vi "Facade.vi"(0 "Data In":T7, 2 "Display State In":T4, 3 "Container State":T6) -> (6 "Data Out":T7, 7 "Display State Out":T4, 8 "Action":T3)   [LabVIEW 2017, in "3D Pie.xctl"]
uses:
  <vilib>/Math Plots/3D Math Plots/3D Pie/3D Pie XCtrl/3D Pie.xctl
  <vilib>/Math Plots/3D Math Plots/3D Pie/3D Pie XCtrl/Data.ctl
  <vilib>/Math Plots/3D Math Plots/3D Plot/3D Plot Datatype/3D Plot Datatype.lvclass
  <vilib>/_xctls/Container State.ctl
  <vilib>/Math Plots/3D Math Plots/3D Pie/3D Pie XCtrl/State.ctl
  <vilib>/Math Plots/3D Math Plots/3D Pie/3D Pie/3D Pie.lvclass
  e:/builds/penguin/labview/branches/2017/dev/dist/vi.lib/Math Plots/3D Math Plots/3D Plot/3D Plot/3D Plot.lvclass
  <vilib>/Math Plots/3D Math Plots/3D Plot/Action String/3DMathPlot Ctrl Act Queue.ctl
  <vilib>/Math Plots/3D Math Plots/3D Plot/Action String/3DMathPlot Ctrl Act Cluster.ctl
  <vilib>/Math Plots/3D Math Plots/3D Plot/Action String/3DMathPlot State Class.ctl
  <vilib>/_xctls/Action.ctl
  <vilib>/Math Plots/3D Math Plots/3D Plot/3D Plot/Typedef/Plot Action.ctl
  <vilib>/Math Plots/3D Math Plots/3D Plot/Action String/3DMathPlot Action String.ctl
  <vilib>/_xctls/XControlSupport.lvlib
  <vilib>/Math Plots/3D Math Plots/3D Plot/3D Plot/3D Plot.lvclass
panel:
  in  "Color Ramp Palette":T1 {"Active Plot" items=["Plot-1"]}
  out "3D Picture Control":refnum<vi>(3d-picture)
  out "Export Image":picture
  out "XY Graph":cluster{dbl, dbl}[](graph)
  out "Render Window":refnum<vi>
  in  "Projection Palette":T2
  out "Intensity Graph":dbl[][](graph)
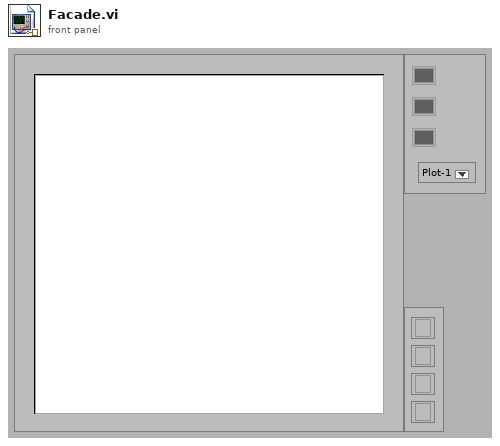
[diagram p1: front panel]
types:
  T1 = cluster{"Active Plot":i32, "Color Pair Array":cluster{"Color Box":u32, "String":string}[]}
  T2 = cluster{"XY Projection":bool, "XZ Projection":bool, "YZ Projection":bool, "3D Projection":bool}
  T3 = typedef "XControlSupport.lvlib/Action.ctl" = cluster{"Data Changed?":bool, "State Changed?":bool, "Action Name":string}
  T4 = typedef "3D Pie.xctl/State.ctl" = cluster{"3D Pie.lvclass":refnum<class "3D Pie.lvclass">, "Control Ref Queue":T5, "Plot Width":u32, "Main Frame Color":u32, "Ramp Palette Color":u32, "Projection Palette Color":u32}
  T5 = typedef "3DMathPlot Ctrl Act Queue.ctl" = refnum<queue>
  T6 = typedef "XControlSupport.lvlib/Container State.ctl" = cluster{"Indicator?":bool, "Run Mode?":bool, " Refnum":refnum<vi>}
  T7 = typedef "3D Pie.xctl/Data.ctl" = refnum<class "3D Plot Datatype.lvclass">[]
  T8 = typedef "3DMathPlot Ctrl Act Cluster.ctl" = cluster{"3D Picture Control":refnum<vi>, "Render Window Refnum":refnum<vi>, "XY Graph":refnum<vi>, "Intensity Graph":refnum<vi>, "Color Legend Palette":refnum<vi>, "Projection Palette":refnum<vi>, "XControl  Ref":refnum<vi>, "Facade Ref":refnum<vi>, "Export Image Ref":refnum<vi>, "Clear Data Flag":bool, "Display State Change Class":T9}
  T9 = typedef "3DMathPlot State Class.ctl" = enum16{"Update All Objects (Undo)", "Update Light Object Only", "Update Axis Object Only", "Update Plot Object Only", "Update Cursor Object Only", "Update Axis Plot Cursor Objects", "No Update"}
  T10 = typedef "3D Plot.lvclass/Actual Transform.ctl" = cluster{"Scale Cluster":cluster{"X Scale":sgl, "Y Scale":sgl, "Z Scale":sgl}, "Translate Cluster":cluster{"X Translate":sgl, "Y Translate":sgl, "Z Translate":sgl}, "Actual Range":T11}
  T11 = typedef "3D Plot.lvclass/Range Clusters.ctl" = cluster{"X Range":cluster{"Max X":sgl, "Min X":sgl}, "Y Range":cluster{"Max Y":sgl, "Min Y":sgl}, "Z Range":cluster{"Max Z":sgl, "Min Z":sgl}}
  T12 = typedef "3D Plot.lvclass/Plot Action.ctl" = cluster{"Light Action":enum16{"Update", "Remove", "Nothing"}, "Axis Action":enum16{"Update", "Remove", "Nothing"}, "Plot Action":enum16{"Update", "Remove", "Nothing"}, "Cursor Action":enum16{"Update", "Remove", "Nothing"}, "Fast Draw Action":enum16{"Update", "Remove", "Nothing"}}
  T13 = enum32{"Towards X-Y Plane", "Towards X-Z Plane", "Towards Y-Z Plane", "User Defined"}
  T14 = typedef "3D Plot.lvclass/Multiplot Representation.ctl" = cluster{"Plot Represention Array":T15[], "Max Range":T11}
  T15 = typedef "3D Plot.lvclass/Plot Representation.ctl" = cluster{"Plot ID":i32, "Plot Range":T11, "Mesh Data":T16, "Dimension":cluster{"X Dimension":i32, "Y Dimension":i32}, "Ramp Range":T11}
  T16 = typedef "3D Plot.lvclass/Mesh Data.ctl" = cluster{"Index Array":u32[], "Vertex Array":cluster{"X":sgl, "Y":sgl, "Z":sgl}[], "Normal Array":cluster{"X":sgl, "Y":sgl, "Z":sgl}[], "Color Index Array":i32[]}
  T17 = typedef "3D Plot.lvclass/Object Cluster.ctl" = cluster{"Root Scene Object":refnum<vi>, "Fast Root Scene Object":refnum<vi>}
  T18 = typedef "3DMathPlot Action String.ctl" = u16
  T19 = typedef "3D Plot.lvclass/Property Cluster.ctl" = cluster{"Graph Property":T20, "Light Property":T24, "Axis Property":T26, "Value Pair Property":T32, "Format Property":T34, "Cursor Property Array":T35, "Appearance Property":T44}
  T20 = typedef "3D Plot.lvclass/Graph Property.ctl" = cluster{"General Property":T21, "View Property":T22, "Grid Plane":T23}
  T21 = typedef "3D Plot.lvclass/General Property.ctl" = cluster{"Plot Area Color":u32, "Fast Draw?":bool, "Clip Data?":bool}
  T22 = typedef "3D Plot.lvclass/View Property.ctl" = cluster{"Projection Mode":enum16{"Orthographic", "Perspective"}, "View Direction":enum32{"Towards X-Y Plane", "Towards X-Z Plane", "Towards Y-Z Plane", "User Defined"}, "User Defined View Direction":cluster{"View Latitude":sgl, "View Longitude":sgl, "View Distance":sgl}}
  T23 = typedef "3D Plot.lvclass/Grid Plane.ctl" = cluster{"Grid Plane Visible":cluster{"Draw Grid Plane X-Y":bool, "Draw Grid Plane Y-Z":bool, "Draw Grid Plane X-Z":bool}, "Grid Antialiasing":bool, "Grid Frame Color":u32}
  T24 = typedef "3D Plot.lvclass/Light Property.ctl" = cluster{"Enable Lighting?":bool, "Ambient Color":u32, "Light Array":T25[]}
  T25 = typedef "3D Plot.lvclass/Light Specific.ctl" = cluster{"Enable Light?":bool, "Light Color":u32, "Light Latitude":sgl, "Light Longitude":sgl, "Light Distance":sgl, "Attenuation":enum16{"None", "Linear", "Quadratic"}}
  T26 = typedef "3D Plot.lvclass/Axis Property.ctl" = cluster{"Caption Property":T27, "Label Property":T28, "Range Property":T29, "Grid Property":T30, "Ticks Property":T31}
  T27 = typedef "3D Plot.lvclass/Caption Property.ctl" = cluster{"Show Caption":cluster{"Show Normal X Caption":bool, "Show Normal Y Caption":bool, "Show Normal Z Caption":bool, "Show Opposite X Caption":bool, "Show Opposite Y Caption":bool, "Show Opposite Z Caption":bool}, "Caption Color":cluster{"Caption Color X":u32, "Caption Color Y":u32, "Caption Color Z":u32}, "Caption Size":cluster{"Caption Size X":u16, "Caption Size Y":u16, "Caption Size Z":u16}, "Caption String":cluster{"Caption X":string, "Caption Y":string, "Caption Z ":string}}
  T28 = typedef "3D Plot.lvclass/Label Property.ctl" = cluster{"Show Label":cluster{"Show Normal X Label":bool, "Show Normal Y Label":bool, "Show Normal Z Label":bool, "Show Opposite X Label":bool, "Show Opposite Y Label":bool, "Show Opposite Z Label":bool}, "Label Color":cluster{"Label Color X":u32, "Label Color Y":u32, "Label Color Z":u32}, "Label Size":cluster{"Label Size X":u16, "Label Size Y":u16, "Labe Size Z":u16}}
  T29 = typedef "3D Plot.lvclass/Range Property.ctl" = cluster{"Range Cluster":T11, "Auto Range":cluster{"Auto Range X":bool, "Auto Range Y":bool, "Auto Range Z":bool}, "Inverted":cluster{"Inverted X":bool, "Inverted Y":bool, "Inverted Z":bool}, "Logarithm":cluster{"Logarithm X":bool, "Logarithm Y":bool, "Logarithm Z":bool}}
  T30 = typedef "3D Plot.lvclass/Grid Property.ctl" = cluster{"Major Grid Visible":cluster{"Draw Major Grid X":bool, "Draw Major Grid Y":bool, "Draw Major Grid Z":bool}, "Major Grid Color":cluster{"Major Grid Color X":u32, "Major Grid Color Y":u32, "Major Grid Color Z":u32}, "Minor Grid Visible":cluster{"Draw Minor Grid X":bool, "Draw Minor Grid Y":bool, "Draw Minor Grid Z":bool}, "Minor Grid Color":cluster{"Minor Grid Color X":u32, "Minor Grid Color Y":u32, "Minor Grid Color Z":u32}}
  T31 = typedef "3D Plot.lvclass/Tick Property.ctl" = cluster{"Major Tick Visible":cluster{"Draw Major Tick X":bool, "Draw Major Tick Y":bool, "Draw Major Tick Z":bool}, "Major Tick Color":cluster{"Major Tick Color X":u32, "Major Tick Color Y":u32, "Major Tick Color Z":u32}, "Major Count":cluster{"Major Count X":u16, "Major Count Y":u16, "Major Count Z":u16}, "Minor Tick Visible":cluster{"Draw Minor Tick X":bool, "Draw Minor Tick Y":bool, "Draw Minor Tick Z":bool}, "Minor Tick Color":cluster{"Minor Tick Color X":u32, "Minor Tick Color Y":u32, "Minor Tick Color Z":u32}, "Minor Count":cluster{"Minor Count X":u16, "Minor Count Y":u16, "Minor Count Z":u16}}
  T32 = typedef "3D Plot.lvclass/Value Pair Property.ctl" = T33[]
  T33 = typedef "3D Plot.lvclass/Value Pair Cluster.ctl" = cluster{"Value Pair Array":cluster{"Value":sgl, "Name":string}[], "Show Tick":bool, "Show Grid":bool, " Label Mode":enum16{"Name", "Value", "None"}}
  T34 = typedef "3D Plot.lvclass/Format Property.ctl" = string[]
  T35 = typedef "3D Plot.lvclass/Cursor Property Array.ctl" = T36[]
  T36 = typedef "3D Plot.lvclass/Cursor Property.ctl" = cluster{"Cursor Visible":bool, "Cursor Enable":bool, "Cursor Position":T37, "Cursor Point":T38, "Cursor Line":T40, "Cursor Plane":T42, "Cursor Text":T43}
  T37 = typedef "3D Plot.lvclass/Cursor Position.ctl" = cluster{"Cursor Plot ID":i32, "Cursor X":sgl, "Cursor Y":sgl, "Cursor Z":sgl, "Cursor Snap To":enum16{"Fixed", "Nearest Plot", "Snap to Plot"}}
  T38 = typedef "3D Plot.lvclass/Cursor Point.ctl" = cluster{"Cursor Point Color":u32, "Cursor Point Size":sgl, "Cursor Point Style":T39}
  T39 = typedef "3D Plot.lvclass/Sprite Type.ctl" = enum16{"None", "Empty Square", "Solid Square", "Empty Diamond", "Solid Diamond", "Empty Circle", "Solid Circle", "Asterisk", "Bold X", "Wireframe Sphere", "Solid Sphere", "Wireframe Cube", "Solid Cube"}
  T40 = typedef "3D Plot.lvclass/Cursor Line.ctl" = cluster{"Cursor Line Color":u32, "Cursor Line Width":sgl, "Cursor Line Style":T41}
  T41 = typedef "3D Plot.lvclass/Line Type.ctl" = enum16{"None", "Solid", "Dash", "Dot", "Dash Dot"}
  T42 = typedef "3D Plot.lvclass/Cursor Plane.ctl" = cluster{"Cursor Plane Color":u32, "Cursor Plane Opacity":sgl, "Draw Cursor Plane X-Z":bool, "Draw Cursor Plane Y-Z":bool, "Draw Cursor Plane X-Y":bool}
  T43 = typedef "3D Plot.lvclass/Cursor Text.ctl" = cluster{"Cursor Text":string, "Cursor Text Size":u16, "Cursor Show Position":bool, "Cursor Show Name":bool, "Cursor Text Color":u32, "Background Color":u32, "Background Opacity":sgl}
  T44 = typedef "3D Plot.lvclass/Apearance Property.ctl" = cluster{"Visibility":T45, "Active Index":cluster{"Active Plot":i32, "Active Cursor":i32, "Active Axis":enum16{"X-axis", "Y-axis", "Z-axis"}, "Active Value Pair":enum16{"X-axis", "Y-axis", "Z-axis"}, "Active Light":enum16{"Light 0", "Light 1", "Light 2", "Light 3"}}, "Backup Data":cluster{"Plot Name":string[]}}
  T45 = typedef "3D Plot.lvclass/Item Visibility.ctl" = cluster{"Projection Palette":bool, "Color Ramp Palette":bool}
  T46 = typedef "LVPoint32TypeDef.ctl" = cluster{"Horizontal":i32, "Vertical":i32}
  T47 = typedef "LVRangeTypeDef.ctl" = cluster{"Minimum":dbl, "Maximum":dbl, "Increment":dbl, "Minor Increment":dbl, "Start":dbl}
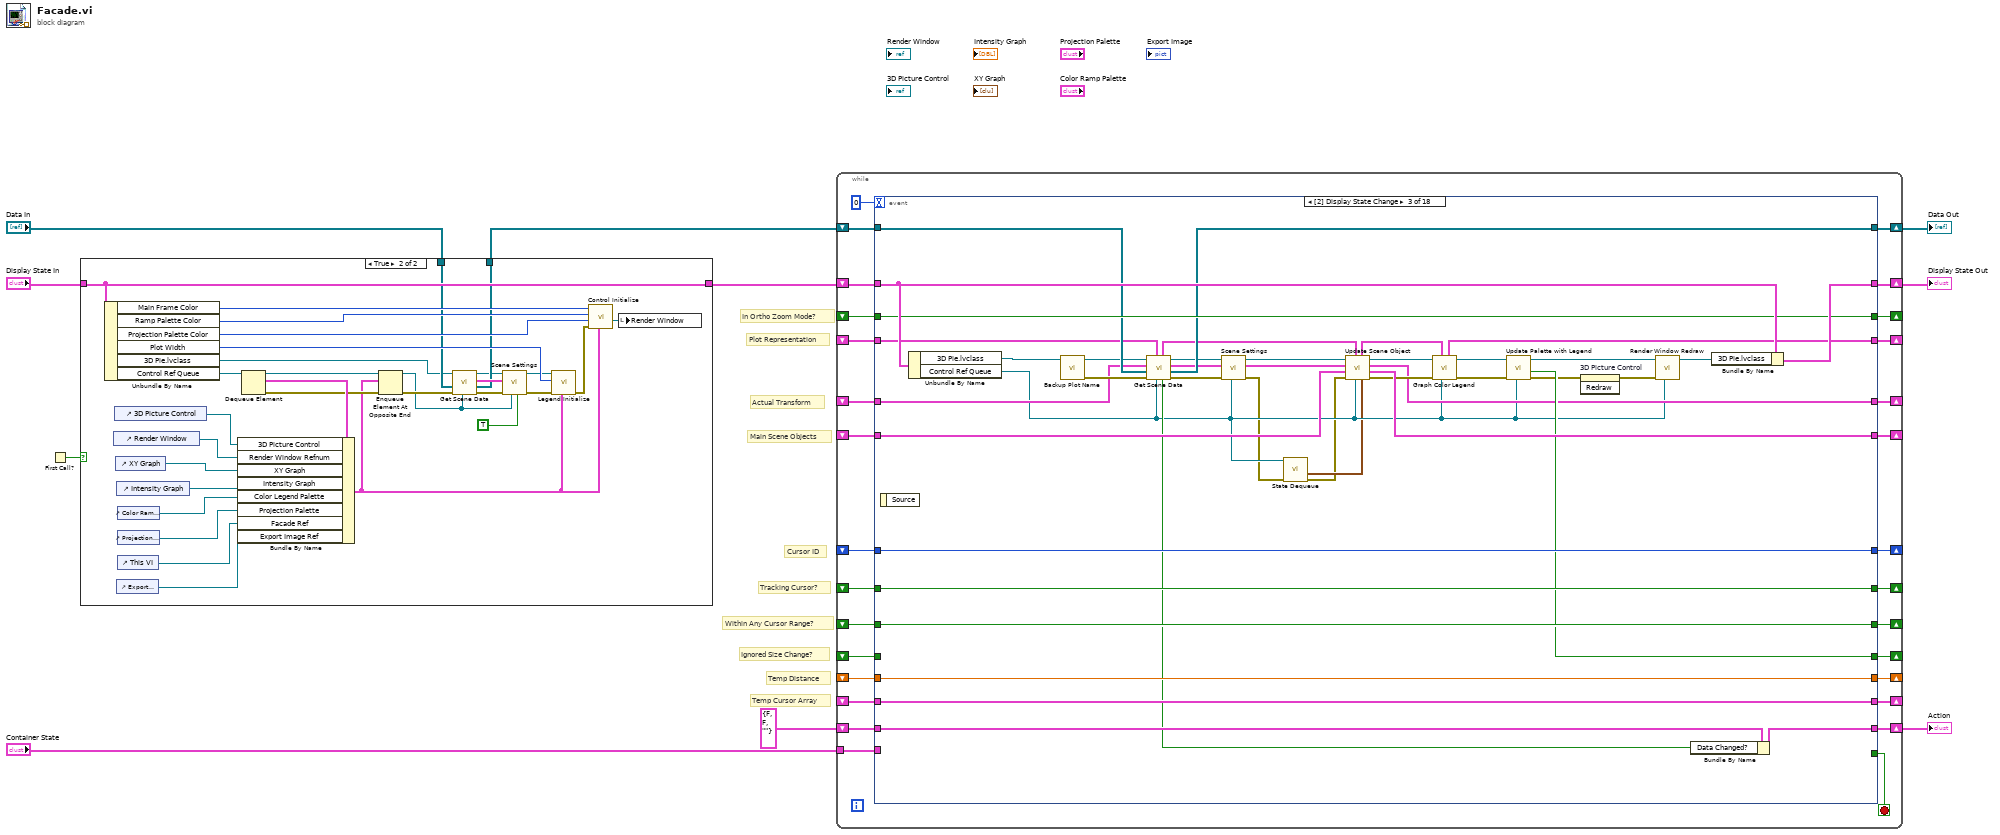
[diagram p0: block diagram]
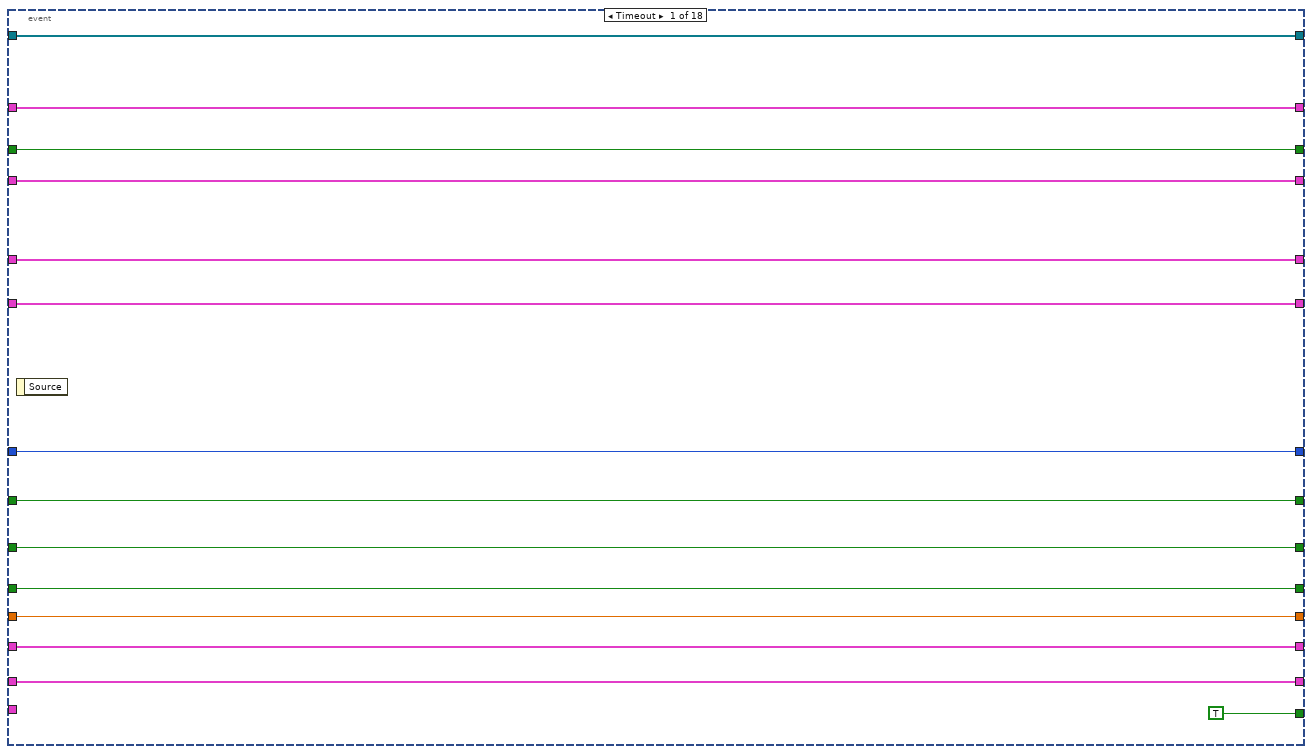
[diagram p2: hidden frame]
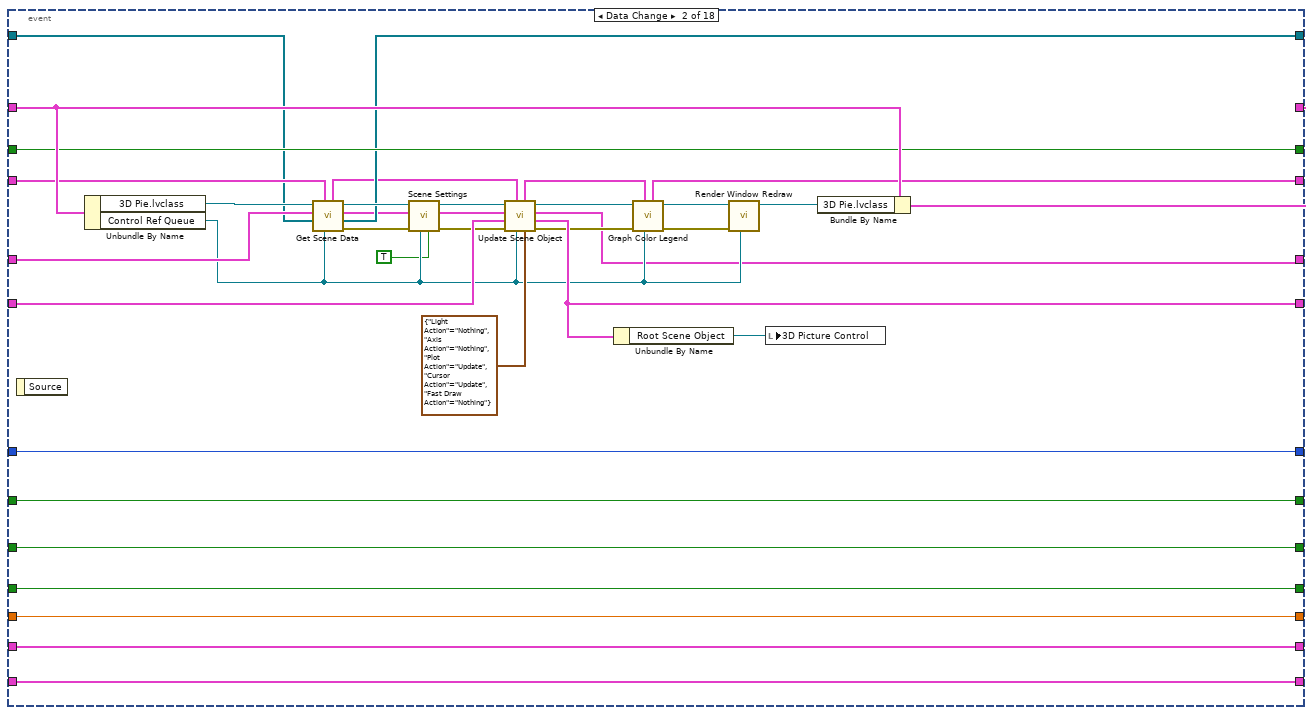
[diagram p3: hidden frame]
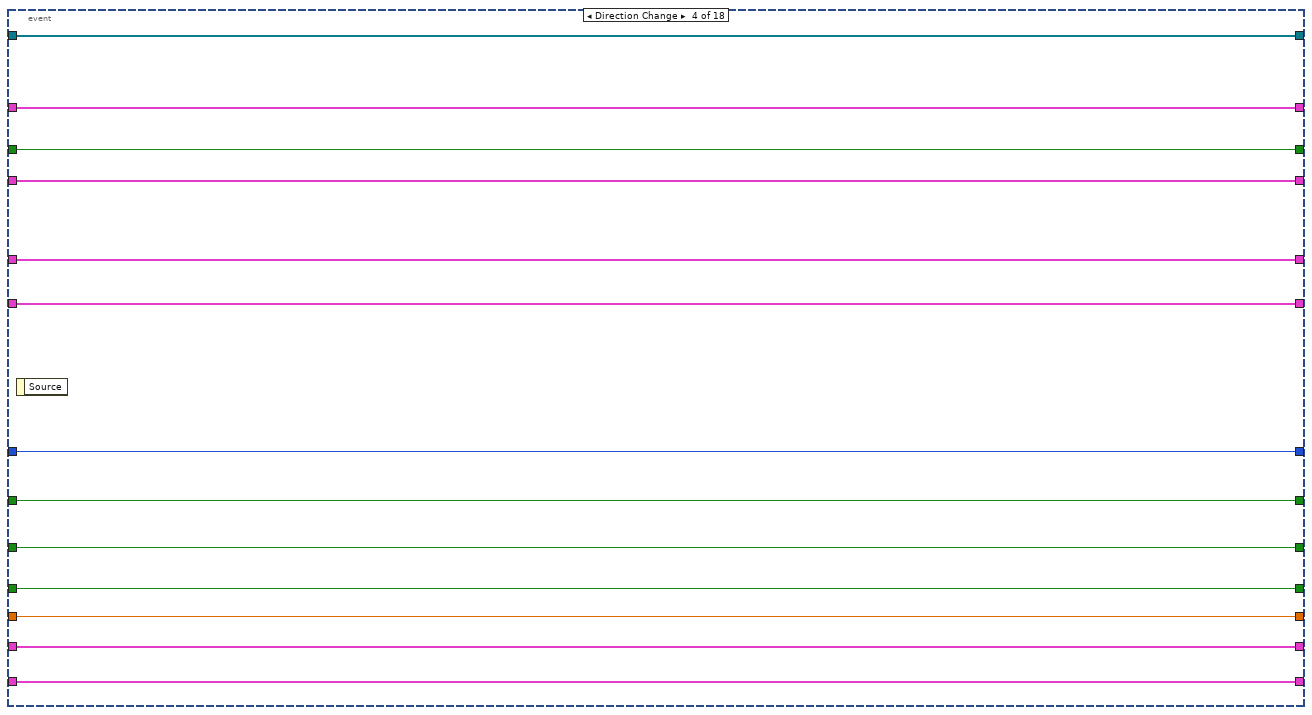
[diagram p4: hidden frame]
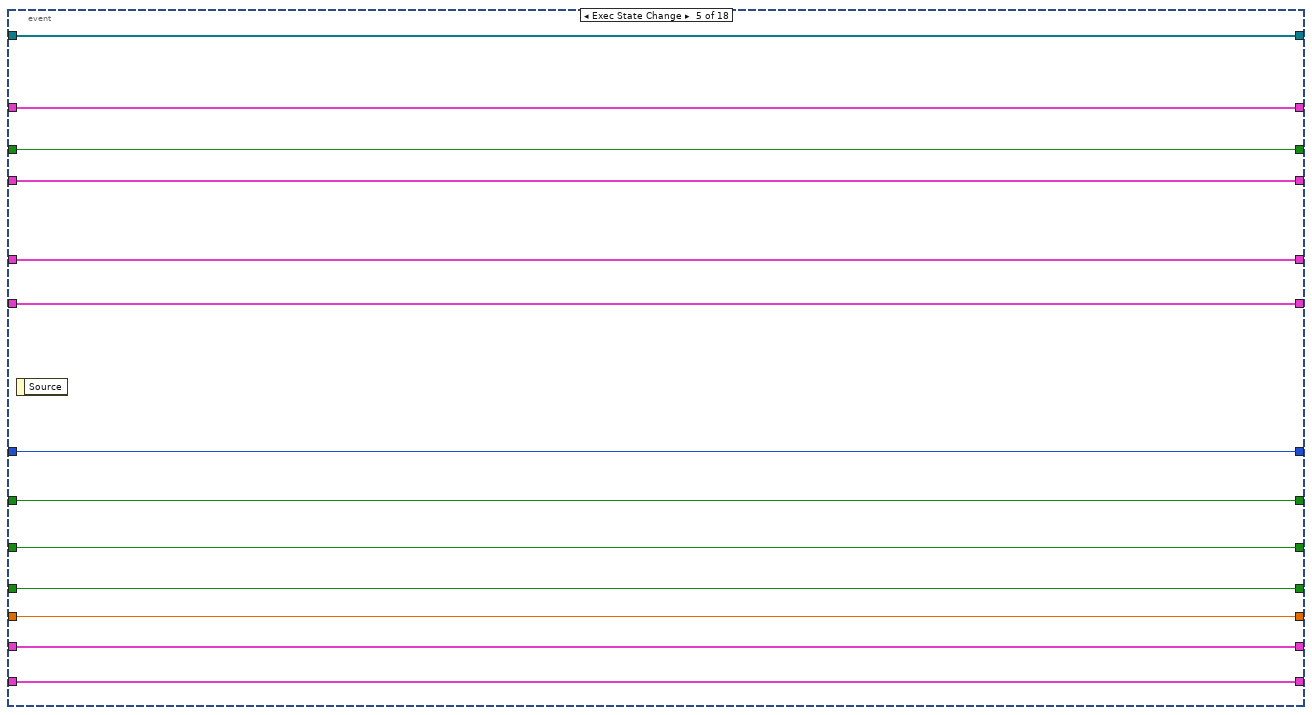
[diagram p5: hidden frame]
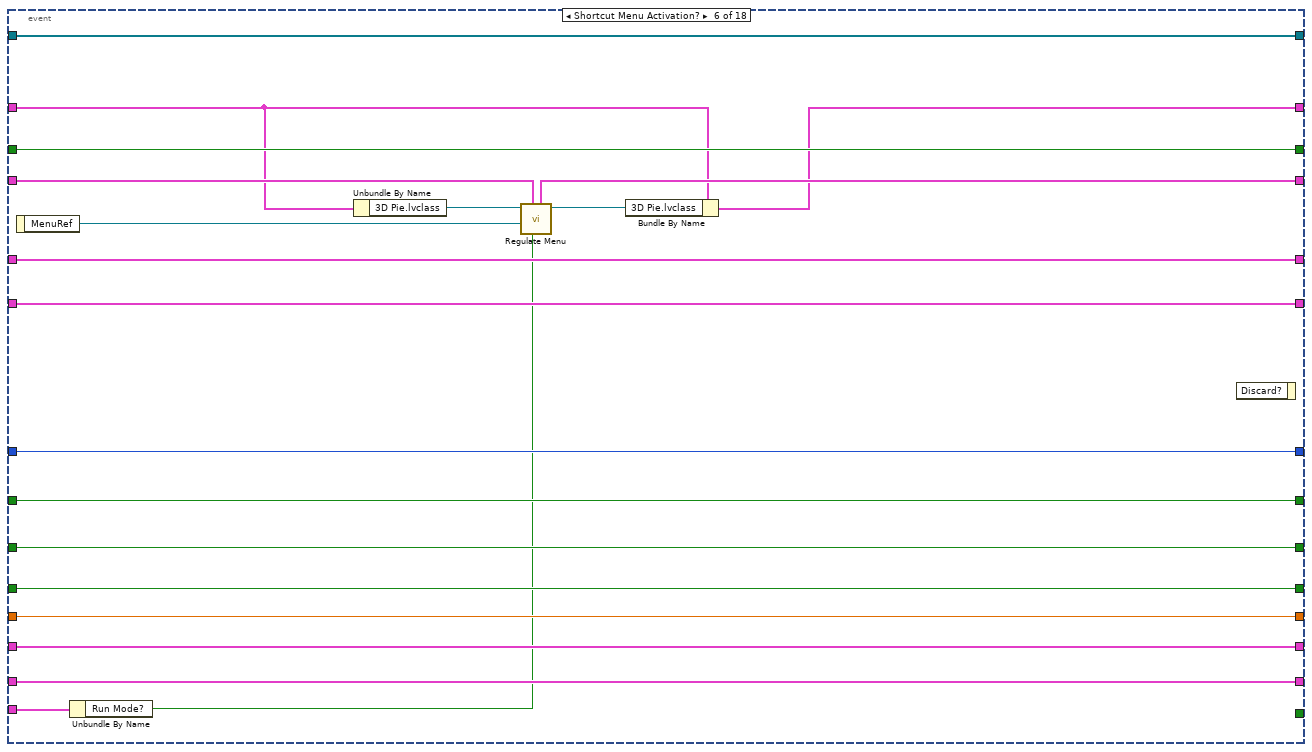
[diagram p6: hidden frame]
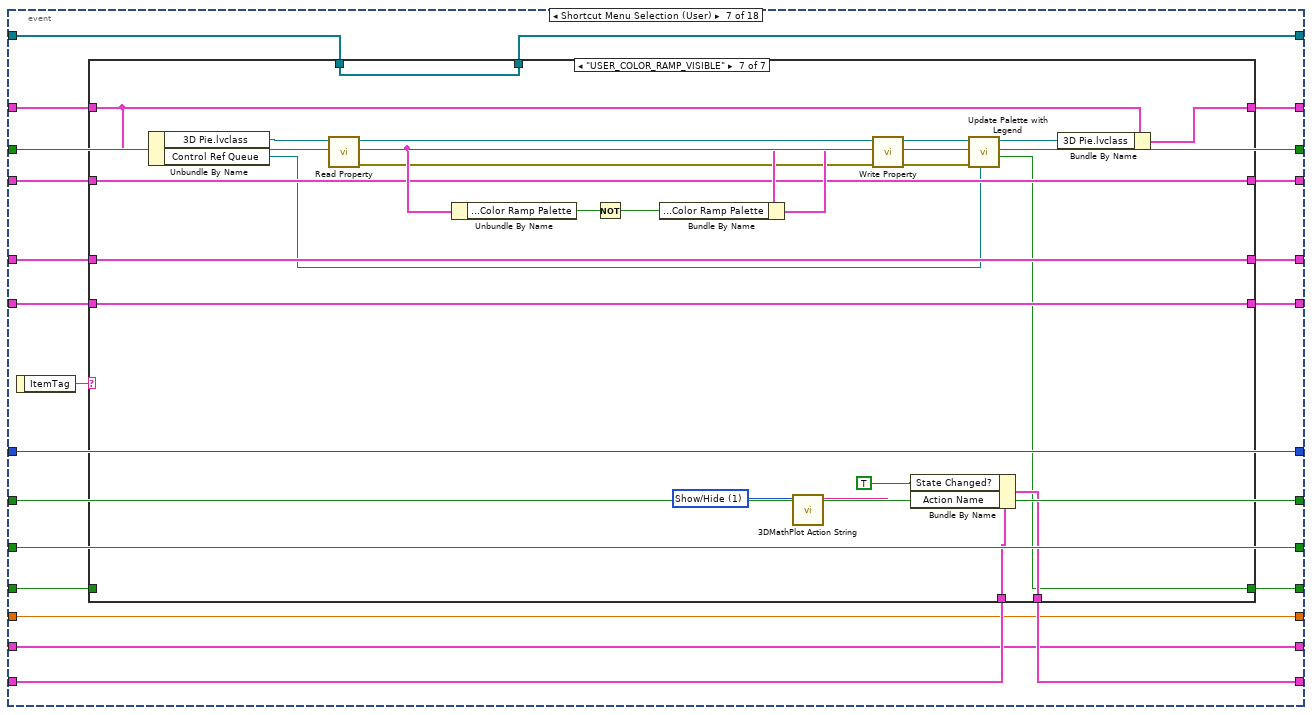
[diagram p7: hidden frame]
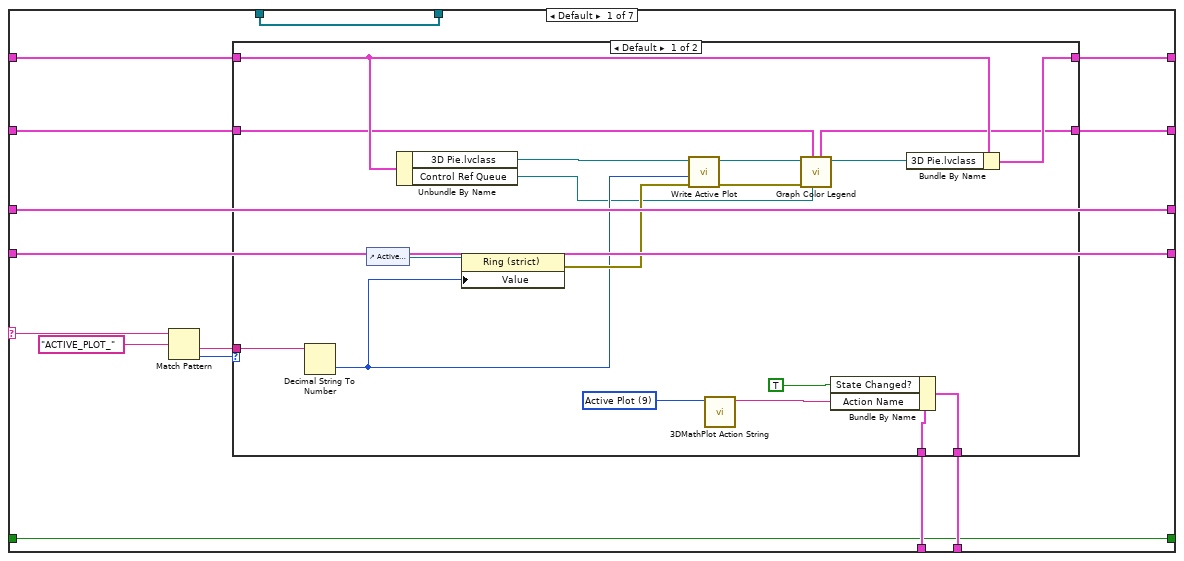
[diagram p8: hidden frame]
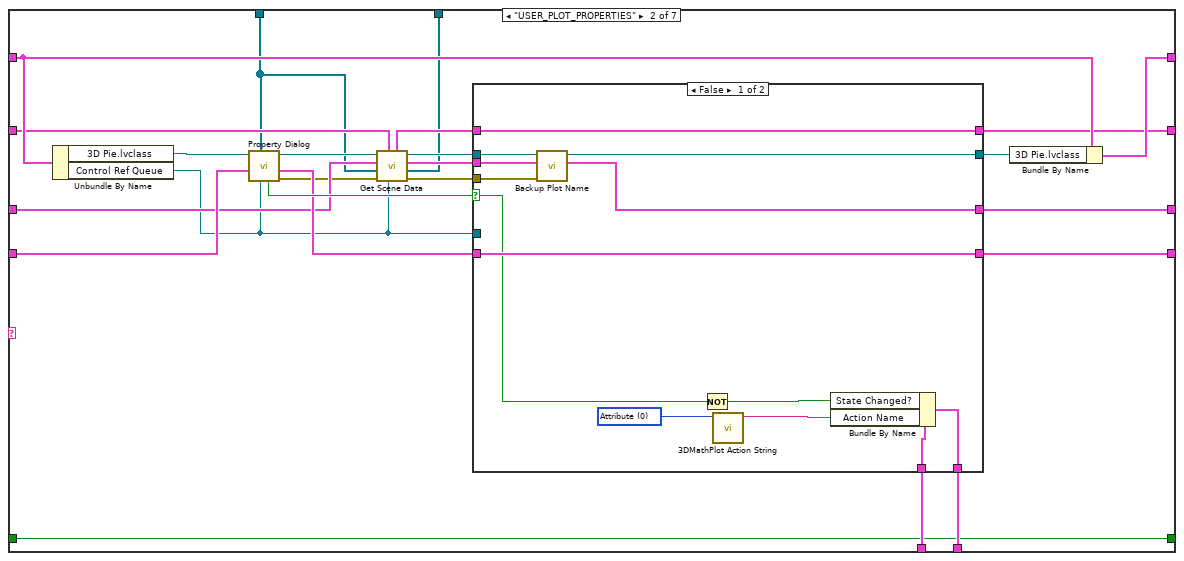
[diagram p10: hidden frame]
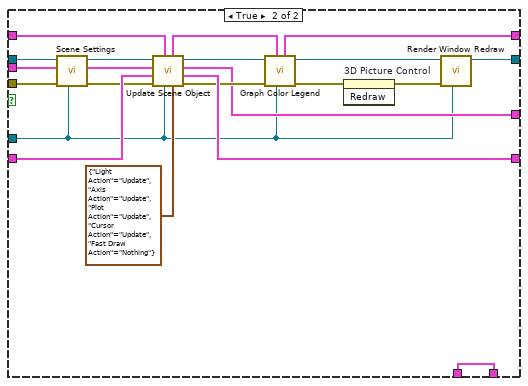
[diagram p11: hidden frame]
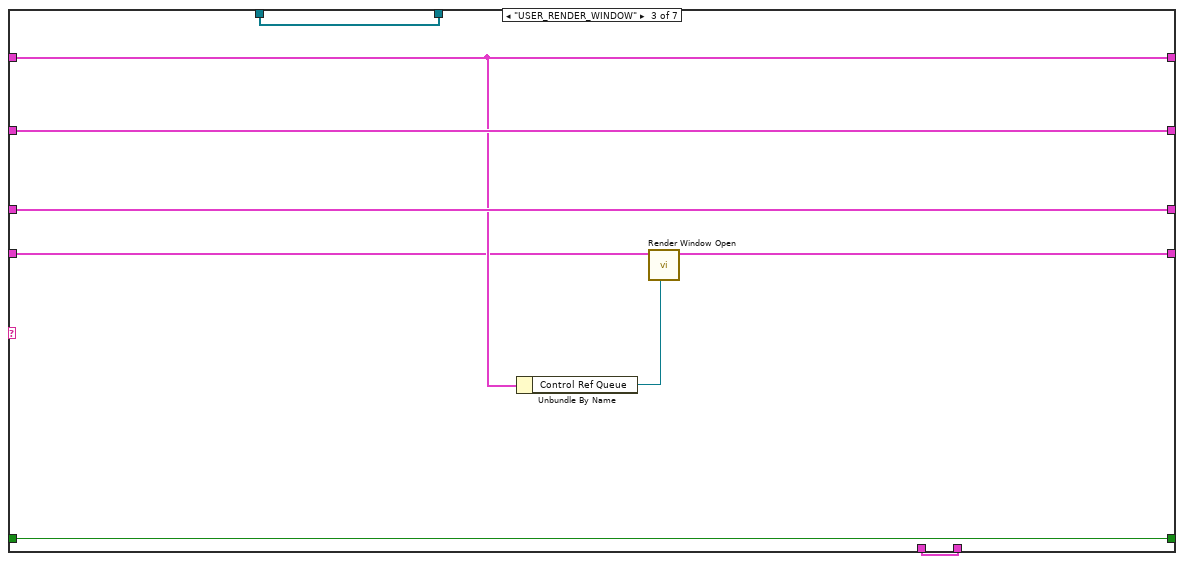
[diagram p12: hidden frame]
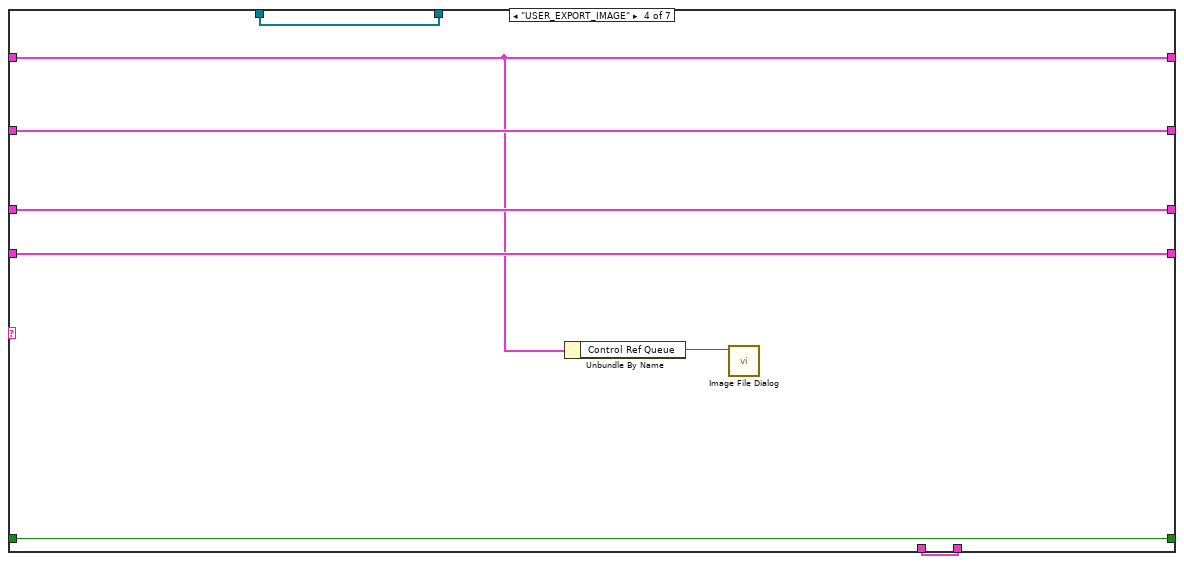
[diagram p13: hidden frame]
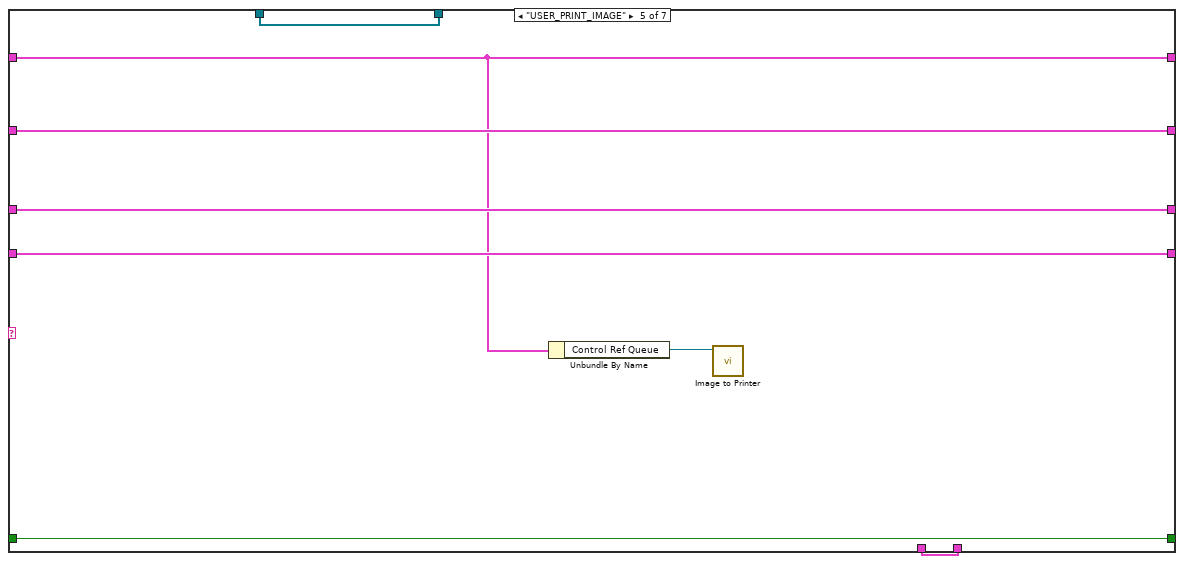
[diagram p14: hidden frame]
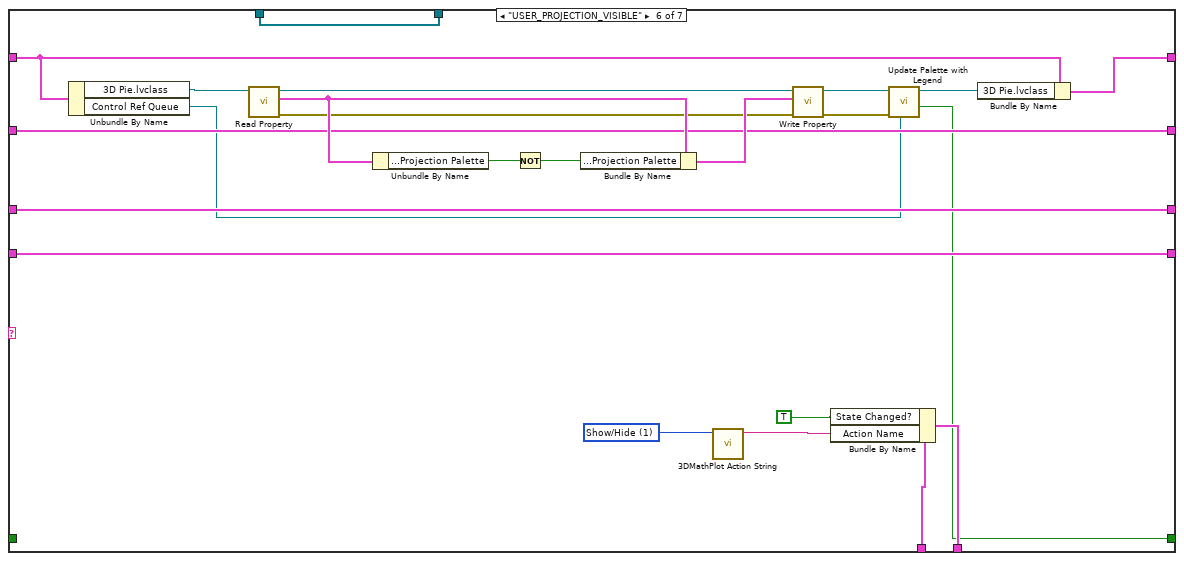
[diagram p15: hidden frame]
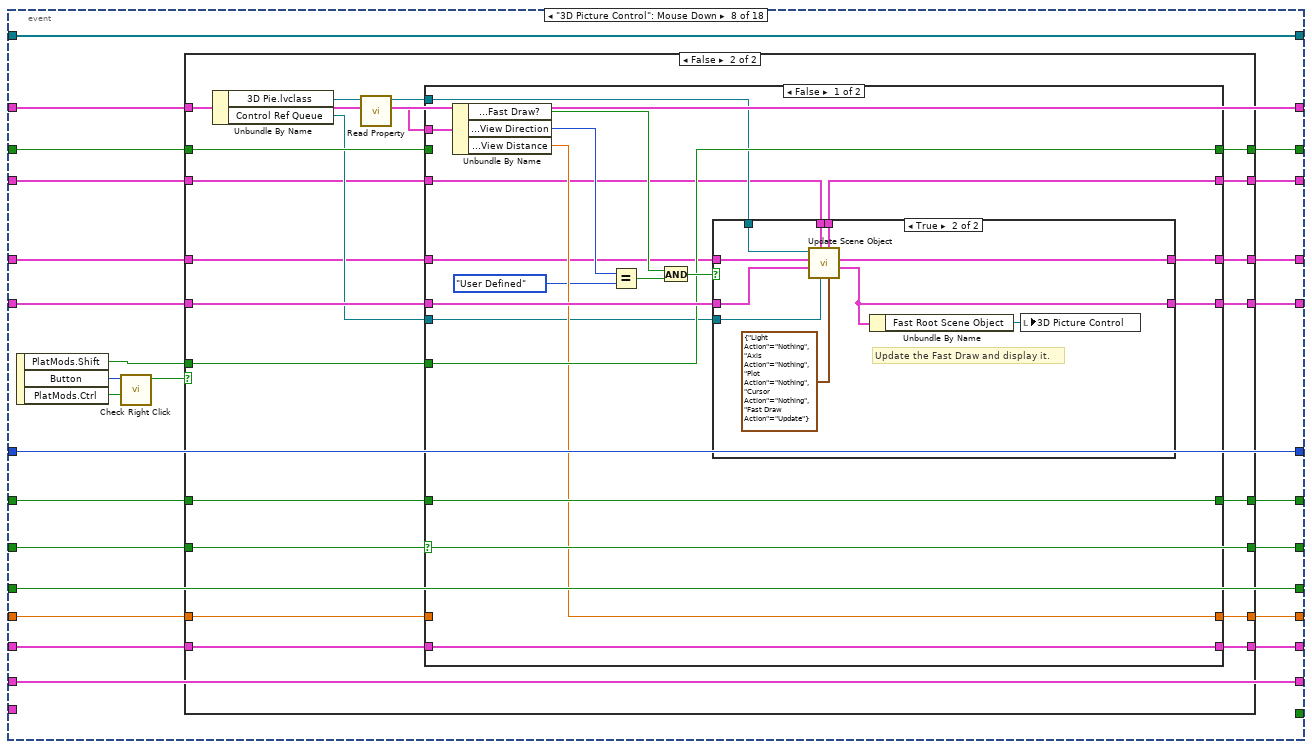
[diagram p16: hidden frame]
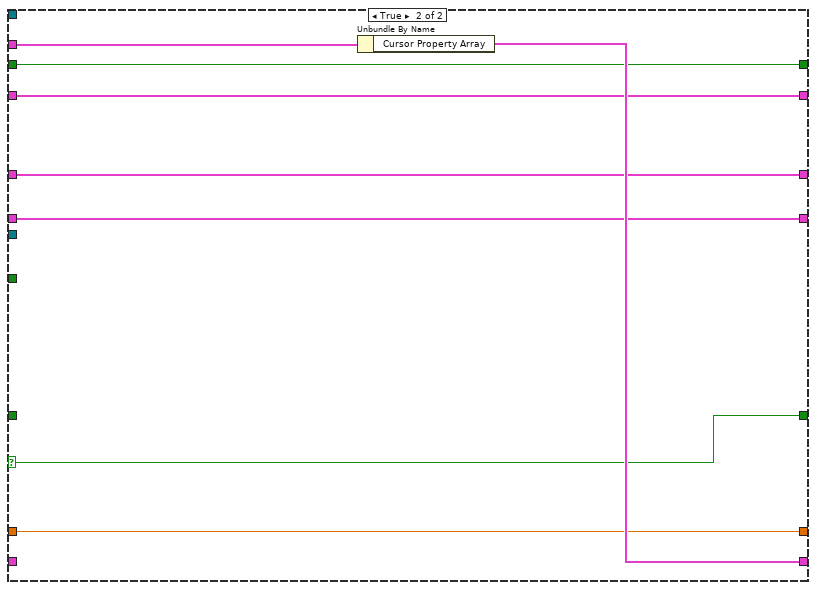
[diagram p19: hidden frame]
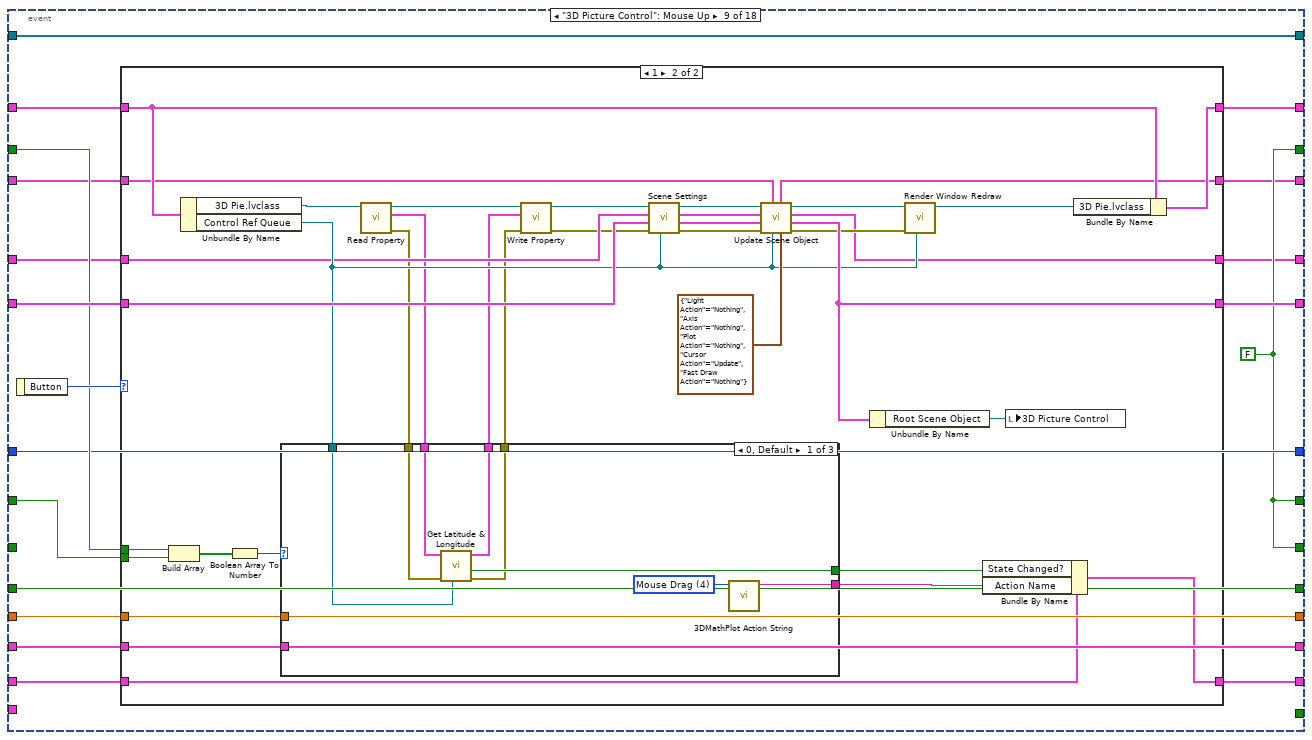
[diagram p20: hidden frame]
diagram:
  # "Ignored Size Change?"
  # "Actual Transform"
  # "Temp Cursor Array"
  # "Temp Distance"
  # "Within Any Cursor Range?"
  # "Tracking Cursor?"
  # "Cursor ID"
  # "Plot Representation"
  # "In Ortho Zoom Mode?"
  # "Main Scene Objects"
  n1 = First Call?() -> (First Call?: T/F=w10:bool)
  n2 = case shown="True" w10 {
    tunnel: "Display State In" -> [w12 w32]
    tunnel: [w12 w32] -> w8
    tunnel: "Data In" -> [w11 w18]
    tunnel: [w11 w17] -> w1
    frame False {
    }
    frame True {
      n3 = Unbundle By Name(w32) -> ("Main Frame Color"=w27:u32, "Ramp Palette Color"=w26:u32, "Projection Palette Color"=w25:u32, "Plot Width"=w23:u32, "3D Pie.lvclass"=w16:refnum<class "3D Pie.lvclass">, "Control Ref Queue"=w31:T5)
      n4 = control-ref of="Render Window"() -> (w37:refnum<vi>)
      n5 = control-ref of="3D Picture Control"() -> (w38:refnum<vi>)
      n6 = control-ref of="XY Graph"() -> (w36:refnum<vi>)
      n7 = control-ref of="Intensity Graph"() -> (w35:refnum<vi>)
      n8 = control-ref of="Export Image"() -> (w30:refnum<vi>)
      n9 = control-ref of="Color Ramp Palette"() -> (w34:refnum<vi>)
      n10 = control-ref of="Projection Palette"() -> (w33:refnum<vi>)
      n11 = control-ref of="This VI"() -> (w42:refnum<vi>)
      n12 = Dequeue Element(queue=w31) -> (queue out=w40:T5, element=w41:T8, error out=w39:errorcluster)  [unwired: 1 in, 2 out]
      n13 = Bundle By Name(cluster=w41, "3D Picture Control"=w38, "Render Window Refnum"=w37, "XY Graph"=w36, "Intensity Graph"=w35, "Color Legend Palette"=w34, "Projection Palette"=w33, "Facade Ref"=w42, "Export Image Ref"=w30) -> (w28:T8)
      n14 = Enqueue Element At Opposite End(queue=w40, element=w28, error in (no error)=w39) -> (queue out=w20:T5, error out=w22:errorcluster)  [unwired: 2 out]
      n15 = call <vilib>:"Get Scene Data.vi"("Control Ref Queue"=w20, "error in (no error)"=w22, "Data In"=w18, "3D Plot.lvclass in"=w16) -> ("error out"=w13:errorcluster, "Data Out"=w17:refnum<class "3D Plot Datatype.lvclass">[], "Actual Transform Out"=w24:T10, "3D Plot.lvclass out"=w15:refnum<class "3D Pie.lvclass">)  [unwired: 2 in, 2 out]
      n16 = call <vilib>:"Scene Settings.vi"("Data Change Event?"=TRUE, "Control Ref Queue"=w20, "error in (no error)"=w13, "Actual Transform In"=w24, "3D Plot.lvclass in"=w15) -> ("error out"=w21:errorcluster, "3D Plot.lvclass out"=w14:refnum<class "3D Pie.lvclass">)  [unwired: 2 in, 3 out]
      n17 = call <vilib>:"Legend Initialize.vi"("Control Ref Cluster"=w28, "error in (no error)"=w21, "XY Plot Width"=w23, "3D Plot.lvclass"=w14) -> ("error out"=w29:errorcluster)  [unwired: 7 out]
      n18 = call <vilib>:"Control Initialize.vi"("Control Ref Cluster"=w28, "error in (no error)"=w29, "Projection Palette Color"=w25, "Ramp Palette Color"=w26, "Main Frame Color"=w27) -> ("New Window Refnum"=w43:refnum<vi>)  [unwired: 6 out]
      n19 = local write "Render Window"(w43) -> ()
    }
  }
  n20 = while {
    shift-right: [w71] -> w4
    shift-left: w8 -> [w72]
    tunnel: "Container State" -> [w68]
    shift-right: [w67] -> w5
    shift-left: w1 -> [w62]
    shift-right: [w65] -> w3
    shift-left: T3 {"Data Changed?"=FALSE, "State Changed?"=FALSE, "Action Name"=""} ("Action") -> [w66]
    shift-right: [w64] -> _
    shift-left: _ -> [w63]
    shift-right: [w61] -> _
    shift-left: _ -> [w48]
    shift-right: [w59] -> _
    shift-left: _ -> [w60]
    shift-right: [w58] -> _
    shift-left: _ -> [w57]
    shift-right: [w55] -> _
    shift-left: _ -> [w56]
    shift-right: [w54] -> _
    shift-left: _ -> [w53]
    shift-right: [w52] -> _
    shift-left: _ -> [w51]
    shift-right: [w50] -> _
    shift-left: _ -> [w49]
    shift-right: [w47] -> _
    shift-left: _ -> [w46]
    shift-right: [w45] -> _
    shift-left: _ -> [w44]
    stop <- w70 stop-if-true
    n21 = event shown="[2] Display State Change" {
      selector: _ -> [_ _ _ _ _ _ _ _ _ _ _ _ _ _ _ _ _ _]
      dyn-events: _ -> [_ _ _ _ _ _ _ _ _ _ _ _ _ _ _ _ _ _]
      timeout: 0 -> [_ _ _ _ _ _ _ _ _ _ _ _ _ _ _ _ _ _]
      tunnel: w72 -> [w74 w121 w161 w175 w188 w190 w225 w407 w500 w583 w609 w636 w663 w690 w714 w737 w800 w818]
      tunnel: [w74 w120 w160 w175 w188 w189 w224 w407 w497 w583 w606 w635 w662 w689 w713 w732 w799 w817] -> w71
      tunnel: [TRUE _ _ _ _ _ _ _ _ _ _ _ _ _ _ _ _ _] -> w70
      tunnel: w68 -> [_ _ _ _ _ w198 _ _ _ _ _ _ _ _ _ _ _ _]
      tunnel: w62 -> [w84 w96 w151 w174 w187 w208 w213 w416 w503 w587 w615 w642 w669 w696 w721 w722 w809 w826]
      tunnel: [w84 w95 w152 w174 w187 w208 w212 w416 w503 w587 w615 w642 w669 w696 w721 w722 w809 w826] -> w67
      tunnel: [w85 w111 w140 w173 w186 w206 w226 w415 w498 w586 w607 w633 w660 w687 w707 w735 w796 w824] -> w65
      tunnel: w66 -> [w85 w111 w162 w173 w186 w206 w227 w415 w499 w586 w608 w634 w661 w688 w708 w734 w797 w824]
      tunnel: [w76 w110 w154 w172 w185 w207 w228 w402 w501 w580 w599 w627 w653 w681 w702 w733 w795 w825] -> w64
      tunnel: w63 -> [w76 w113 w155 w172 w185 w207 w229 w411 w502 w581 w599 w627 w653 w681 w702 w738 w794 w825]
      tunnel: [w83 w118 w153 w171 w184 w205 w218 w399 w491 w584 w610 w641 w668 w695 w720 w743 w804 w821] -> w61
      tunnel: w48 -> [w83 w118 w153 w171 w184 w205 w218 w408 w495 w585 w610 w641 w668 w695 w720 w743 w804 w821]
      tunnel: w60 -> [w82 w117 w159 w170 w183 w204 w219 w414 w492 w579 w611 w640 w667 w694 w719 w729 w805 w822]
      tunnel: [w82 w117 w159 w170 w183 w204 w219 w414 w492 w578 w611 w640 w667 w694 w719 w729 w805 w822] -> w59
      tunnel: w57 -> [w81 w116 w158 w169 w182 w203 w220 w406 w494 w575 w612 w639 w666 w693 w718 w728 w806 w823]
      tunnel: [w81 w116 w158 w169 w182 w203 w220 w398 w491 w575 w612 w639 w666 w693 w718 w728 w806 w823] -> w58
      tunnel: w56 -> [w80 w115 w157 w168 w181 w202 w221 w405 _ _ w613 w638 w665 w692 w717 w727 w807 w819]
      tunnel: [w80 w115 w157 w168 w181 w202 w221 w397 w491 w574 w613 w638 w665 w692 w717 w727 w807 w819] -> w55
      tunnel: [w79 w114 w156 w167 w180 w201 w222 w395 w493 w577 w614 w637 w664 w691 w716 w723 w808 w820] -> w54
      tunnel: w53 -> [w79 w114 w156 w167 w180 w201 w222 w403 w493 _ w614 w637 w664 w691 w716 w723 w808 w820]
      tunnel: [w77 w89 w127 w166 w179 w193 w216 w400 w489 w573 w591 w624 w651 w678 w697 w731 w782 w814] -> w52
      tunnel: w51 -> [w77 w98 w133 w166 w179 w194 w217 w409 w490 w573 w591 w624 w651 w678 w698 w736 w778 w814]
      tunnel: w49 -> [w78 w97 w134 w165 w178 w200 w215 w410 w488 w572 w593 w623 w650 w677 w703 w740 w781 w815]
      tunnel: [w78 w88 w128 w165 w178 w200 w214 w401 w487 w572 w592 w622 w649 w676 w703 w730 w783 w815] -> w50
      tunnel: [w75 w107 w147 w164 w177 w199 w211 w413 w486 w571 w603 w630 w657 w684 w705 w724 w791 FALSE] -> w47
      tunnel: w46 -> [w75 w107 _ w164 w177 w199 w210 w413 w486 w571 w603 w630 w657 w684 w705 w726 w791 w811]
      tunnel: [w73 w101 w141 w163 w176 w197 w209 w396 w485 w565 w601 w628 w655 w682 w701 w725 w784 w813] -> w45
      tunnel: w44 -> [w73 w101 w141 w163 w176 w197 w209 w404 w485 _ w601 w628 w655 w682 w701 w725 w784 w813]
      event Timeout {
        n22 = event-data() -> ()  [unwired: 2 out]
      }
      event Data Change {
        n23 = event-data() -> ()  [unwired: 2 out]
        n24 = Unbundle By Name(w121) -> ("3D Pie.lvclass"=w100:refnum<class "3D Pie.lvclass">, "Control Ref Queue"=w92:T5)
        n25 = call <vilib>:"Get Scene Data.vi"("Control Ref Queue"=w92, "Multiplot Representation In"=w98, "Data In"=w96, "Actual Transform In"=w97, "3D Plot.lvclass in"=w100) -> ("error out"=w93:errorcluster, "Data Out"=w95:refnum<class "3D Plot Datatype.lvclass">[], "Actual Transform Out"=w94:T10, "3D Plot.lvclass out"=w99:refnum<class "3D Pie.lvclass">, "Multiplot Representation Out"=w91:T14)  [unwired: 1 in, 1 out]
        n26 = call <vilib>:"Scene Settings.vi"("Data Change Event?"=TRUE, "Control Ref Queue"=w92, "error in (no error)"=w93, "Actual Transform In"=w94, "3D Plot.lvclass in"=w99) -> ("error out"=w102:errorcluster, "Actual Transform Out"=w112:T10, "3D Plot.lvclass out"=w103:refnum<class "3D Pie.lvclass">)  [unwired: 2 in, 2 out]
        n27 = call <vilib>:"Update Scene Object.vi"("Action"=T12 {"Light Action"=enum."Nothing", "Axis Action"=enum."Nothing", "Plot Action"=enum."Update", "Cursor Action"=enum."Update", "Fast Draw Action"=enum."Nothing"}, "Control Ref Queue"=w92, "Multiplot Representation In"=w91, "error in (no error)"=w102, "Object Cluster In"=w113, "Actual Transform In"=w112, "3D Plot.lvclass in"=w103) -> ("error out"=w108:errorcluster, "Object Cluster Out"=w110:T17, "Actual Transform Out"=w88:T10, "3D Plot.lvclass out"=w109:refnum<class "3D Pie.lvclass">, "Multiplot Representation Out"=w90:T14)
        n28 = Unbundle By Name(w110) -> ("Root Scene Object"=w119:refnum<vi>)
        n29 = call-dynamic "Graph Color Legend.vi"("Control Ref Queue"=w92, "Multiplot Representation In"=w90, "error in (no error)"=w108, "3D Pie.lvclass in"=w109) -> ("error out"=w104:errorcluster, "3D Pie.lvclass out"=w105:refnum<class "3D Pie.lvclass">, "Multiplot Representation Out"=w89:T14)  [unwired: 2 in, 3 out]
        n30 = call <vilib>:"Render Window Redraw.vi"("Control Ref Queue"=w92, "error in (no error)"=w104) -> ()  [unwired: 1 in, 9 out]
        n31 = local write "3D Picture Control"(w119) -> ()
        n32 = Bundle By Name(cluster=w121, "3D Pie.lvclass"=w105) -> (w120:T4)
      }
      event Display State Change {
        n33 = event-data() -> ()  [unwired: 2 out]
        n34 = Unbundle By Name(w161) -> ("3D Pie.lvclass"=w126:refnum<class "3D Pie.lvclass">, "Control Ref Queue"=w125:T5)
        n35 = call-dynamic "Backup Plot Name.vi"("3D Pie.lvclass in"=w126) -> ("error out"=w135:errorcluster, "3D Pie.lvclass out"=w138:refnum<class "3D Pie.lvclass">)  [unwired: 1 in, 8 out]
        n36 = call <vilib>:"Get Scene Data.vi"("Control Ref Queue"=w125, "Multiplot Representation In"=w133, "error in (no error)"=w135, "Data In"=w151, "Actual Transform In"=w134, "3D Plot.lvclass in"=w138) -> ("error out"=w137:errorcluster, "Data Out"=w152:refnum<class "3D Plot Datatype.lvclass">[], "Actual Transform Out"=w132:T10, "3D Plot.lvclass out"=w136:refnum<class "3D Pie.lvclass">, "Data Cleaned?"=w139:bool, "Multiplot Representation Out"=w130:T14)
        n37 = call <vilib>:"Scene Settings.vi"("Control Ref Queue"=w125, "error in (no error)"=w137, "Actual Transform In"=w132, "3D Plot.lvclass in"=w136) -> ("error out"=w122:errorcluster, "Actual Transform Out"=w131:T10, "3D Plot.lvclass out"=w142:refnum<class "3D Pie.lvclass">)  [unwired: 3 in, 2 out]
        n38 = call <vilib>:"State Dequeue.vi"("error in (no error)"=w122, "Control Ref Queue"=w125) -> ("error out"=w123:errorcluster, "Action"=w124:T12)  [unwired: 8 out]
        n39 = call <vilib>:"Update Scene Object.vi"("Action"=w124, "Control Ref Queue"=w125, "Multiplot Representation In"=w130, "error in (no error)"=w123, "Object Cluster In"=w155, "Actual Transform In"=w131, "3D Plot.lvclass in"=w142) -> ("error out"=w149:errorcluster, "Object Cluster Out"=w154:T17, "Actual Transform Out"=w128:T10, "3D Plot.lvclass out"=w150:refnum<class "3D Pie.lvclass">, "Multiplot Representation Out"=w129:T14)
        n40 = call-dynamic "Graph Color Legend.vi"("Control Ref Queue"=w125, "Multiplot Representation In"=w129, "error in (no error)"=w149, "3D Pie.lvclass in"=w150) -> ("error out"=w145:errorcluster, "3D Pie.lvclass out"=w146:refnum<class "3D Pie.lvclass">, "Multiplot Representation Out"=w127:T14)  [unwired: 2 in, 3 out]
        n41 = call <vilib>:"Update Palette with Legend.vi"("Control Ref Queue"=w125, "error in (no error)"=w145, "3D Plot.lvclass"=w146) -> ("error out"=w144:errorcluster, "Ignore the size change?"=w147:bool, "3D Plot.lvclass out"=w148:refnum<class "3D Pie.lvclass">)  [unwired: 6 out]
        n42 = invoke on="3D Picture Control" class="SceneGraphDisp (strict)" method="Redraw"(error in=w144) -> (error out=w143:errorcluster)  [unwired: 2 in, 2 out]
        n43 = call <vilib>:"Render Window Redraw.vi"("Control Ref Queue"=w125, "error in (no error)"=w143) -> ()  [unwired: 1 in, 9 out]
        n44 = Bundle By Name(cluster=w162, "Data Changed?"=w139) -> (w140:T3)
        n45 = Bundle By Name(cluster=w161, "3D Pie.lvclass"=w148) -> (w160:T4)
      }
      event Direction Change {
        n46 = event-data() -> ()  [unwired: 2 out]
      }
      event Exec State Change {
        n47 = event-data() -> ()  [unwired: 2 out]
      }
      event Shortcut Menu Activation? {
        n48 = event-data() -> ("MenuRef"=w192:refnum<k9>)  [unwired: 1 out]
        n49 = Unbundle By Name(w198) -> ("Run Mode?"=w191:bool)
        n50 = Unbundle By Name(w190) -> ("3D Pie.lvclass"=w196:refnum<class "3D Pie.lvclass">)
        n51 = call <vilib>:"Regulate Menu.vi"("Run Mode?"=w191, "Multiplot Representation In"=w194, "MenuRef"=w192, "3D Plot.lvclass in"=w196) -> ("3D Plot.lvclass out"=w195:refnum<class "3D Pie.lvclass">, "Multiplot Representation Out"=w193:T14)  [unwired: 3 in, 3 out]
        n52 = Bundle By Name(cluster=w190, "3D Pie.lvclass"=w195) -> (w189:T4)
        n53 = event-data() -> ()  [unwired: 1 in, 2 out]
      }
      event Shortcut Menu Selection (User) {
        n54 = event-data() -> ("ItemTag"=w223:string)  [unwired: 1 out]
        n55 = case shown="\"USER_COLOR_RAMP_VISIBLE\"" w223 {
          selector: w223 -> [w242 _ _ _ _ _ _]
          tunnel: w225 -> [w239 w288 w324 w331 w338 w359 w385]
          tunnel: [w238 w287 w324 w331 w338 w358 w384] -> w224
          tunnel: w229 -> [w243 w278 w322 w337 w345 w364 w383]
          tunnel: [w243 w285 w321 w337 w345 w364 w383] -> w228
          tunnel: w227 -> [w235 w281 w327 w336 w340 w367 w380]
          tunnel: [w236 w280 w327 w336 w340 w366 w379] -> w226
          tunnel: w217 -> [w232 w273 w328 w335 w344 w357 w382]
          tunnel: [w231 w284 w328 w335 w344 w357 w382] -> w216
          tunnel: w215 -> [w230 w271 w325 w332 w343 w356 w381]
          tunnel: [w230 w282 w325 w332 w343 w356 w381] -> w214
          tunnel: w213 -> [w234 w269 w329 w334 w342 w353 w376]
          tunnel: [w234 w268 w329 w334 w342 w353 w376] -> w212
          tunnel: [w233 w279 w326 w333 w339 w347 w370] -> w211
          tunnel: w210 -> [w233 w279 w326 w333 w339 _ _]
          frame Default {
            n56 = Match Pattern(string=w242, regular expression="ACTIVE_PLOT_") -> (after substring=w237:string, offset past match=w240:i32)  [unwired: 3 out]
            n57 = case shown="Default" w240 {
              tunnel: w239 -> [w254 w264]
              tunnel: [w253 w264] -> w238
              tunnel: w237 -> [w260 _]
              tunnel: [w255 w263] -> w236
              tunnel: w235 -> [w256 w263]
              tunnel: w232 -> [w246 w262]
              tunnel: [w245 w262] -> w231
              frame Default {
                w257 = T18 9 items=["Attribute", "Show/Hide", "Cursor Move", "Zoom", "Mouse Drag", "XY Projection", "YZ Projection", "XZ Projection", "3D Projection", "Active Plot", "Scale"] ("Global String")
                n58 = Decimal String To Number(string=w260) -> (number=w251:i32)  [unwired: 3 out]
                n59 = control-ref of="Active Plot"() -> (w244:refnum<vi>)
                n60 = Unbundle By Name(w254) -> ("3D Pie.lvclass"=w261:refnum<class "3D Pie.lvclass">, "Control Ref Queue"=w249:T5)
                n61 = property class="Ring (strict)"(reference=w244, "Value"=w251) -> (error out=w252:errorcluster)  [unwired: 1 in, 1 out]
                n62 = call-dynamic "Write Active Plot.vi"("error in (no error)"=w252, "Active Plot"=w251, "3D Plot.lvclass in"=w261) -> ("error out"=w247:errorcluster, "3D Plot.lvclass out"=w248:refnum<class "3D Pie.lvclass">)  [unwired: 7 in]
                n63 = call <vilib>:"3DMathPlot Action String.vi"("Global String"=w257) -> ("String Out"=w258:string)  [unwired: 10 out]
                n64 = call-dynamic "Graph Color Legend.vi"("Control Ref Queue"=w249, "Multiplot Representation In"=w246, "error in (no error)"=w247, "3D Pie.lvclass in"=w248) -> ("3D Pie.lvclass out"=w250:refnum<class "3D Pie.lvclass">, "Multiplot Representation Out"=w245:T14)  [unwired: 2 in, 4 out]
                n65 = Bundle By Name(cluster=w256, "State Changed?"=TRUE ("Data Changed?"), "Action Name"=w258) -> (w255:T3)
                n66 = Bundle By Name(cluster=w254, "3D Pie.lvclass"=w250) -> (w253:T4)
              }
              frame -1 {
              }
            }
          }
          frame "USER_PLOT_PROPERTIES" {
            n67 = Unbundle By Name(w288) -> ("3D Pie.lvclass"=w286:refnum<class "3D Pie.lvclass">, "Control Ref Queue"=w265:T5)
            n68 = call-dynamic "Property Dialog.vi"("Control Ref Queue"=w265, "Data"=w269, "Object Cluster In"=w278, "3D Pie in"=w286) -> ("error out"=w267:errorcluster, "Object Cluster Out"=w276:T17, "3D Pie out"=w275:refnum<class "3D Pie.lvclass">, "Cancel?"=w277:bool)  [unwired: 1 in, 3 out]
            n69 = call <vilib>:"Get Scene Data.vi"("Control Ref Queue"=w265, "Multiplot Representation In"=w273, "error in (no error)"=w267, "Data In"=w269, "Actual Transform In"=w271, "3D Plot.lvclass in"=w275) -> ("error out"=w266:errorcluster, "Data Out"=w268:refnum<class "3D Plot Datatype.lvclass">[], "Actual Transform Out"=w270:T10, "3D Plot.lvclass out"=w274:refnum<class "3D Pie.lvclass">, "Multiplot Representation Out"=w272:T14)  [unwired: 1 out]
            n70 = case shown="False" w277 {
              selector: w277 -> [w290 _]
              tunnel: w276 -> [w298 w313]
              tunnel: w272 -> [w299 w304]
              tunnel: [w298 w320] -> w285
              tunnel: [w299 w307] -> w284
              tunnel: w274 -> [w293 w302]
              tunnel: w266 -> [w292 w303]
              tunnel: [w291 w317] -> w283
              tunnel: [w300 w306] -> w282
              tunnel: w270 -> [w300 w301]
              tunnel: w281 -> [w295 w314]
              tunnel: [w294 w314] -> w280
              tunnel: w265 -> [_ w305]
              frame False {
                w296 = T18 0 items=["Attribute", "Show/Hide", "Cursor Move", "Zoom", "Mouse Drag", "XY Projection", "YZ Projection", "XZ Projection", "3D Projection", "Active Plot", "Scale"] ("Global String")
                n71 = call-dynamic "Backup Plot Name.vi"("error in (no error)"=w292, "3D Pie.lvclass in"=w293) -> ("3D Pie.lvclass out"=w291:refnum<class "3D Pie.lvclass">)  [unwired: 9 out]
                n72 = Not(x=w290) -> (.not. x?=w289:bool)
                n73 = call <vilib>:"3DMathPlot Action String.vi"("Global String"=w296) -> ("String Out"=w297:string)  [unwired: 10 out]
                n74 = Bundle By Name(cluster=w295, "State Changed?"=w289, "Action Name"=w297) -> (w294:T3)
              }
              frame True {
                n75 = call <vilib>:"Scene Settings.vi"("Control Ref Queue"=w305, "error in (no error)"=w303, "Actual Transform In"=w301, "3D Plot.lvclass in"=w302) -> ("error out"=w309:errorcluster, "Actual Transform Out"=w319:T10, "3D Plot.lvclass out"=w310:refnum<class "3D Pie.lvclass">)  [unwired: 3 in, 2 out]
                n76 = call <vilib>:"Update Scene Object.vi"("Action"=T12 {"Light Action"=enum."Update", "Axis Action"=enum."Update", "Plot Action"=enum."Update", "Cursor Action"=enum."Update", "Fast Draw Action"=enum."Nothing"}, "Control Ref Queue"=w305, "Multiplot Representation In"=w304, "error in (no error)"=w309, "Object Cluster In"=w313, "Actual Transform In"=w319, "3D Plot.lvclass in"=w310) -> ("error out"=w316:errorcluster, "Object Cluster Out"=w320:T17, "Actual Transform Out"=w306:T10, "3D Plot.lvclass out"=w318:refnum<class "3D Pie.lvclass">, "Multiplot Representation Out"=w308:T14)
                n77 = call-dynamic "Graph Color Legend.vi"("Control Ref Queue"=w305, "Multiplot Representation In"=w308, "error in (no error)"=w316, "3D Pie.lvclass in"=w318) -> ("error out"=w312:errorcluster, "3D Pie.lvclass out"=w317:refnum<class "3D Pie.lvclass">, "Multiplot Representation Out"=w307:T14)  [unwired: 2 in, 3 out]
                n78 = invoke on="3D Picture Control" class="SceneGraphDisp (strict)" method="Redraw"(error in=w312) -> (error out=w311:errorcluster)  [unwired: 2 in, 2 out]
                n79 = call <vilib>:"Render Window Redraw.vi"("Control Ref Queue"=w305, "error in (no error)"=w311) -> ()  [unwired: 1 in, 9 out]
              }
            }
            n80 = Bundle By Name(cluster=w288, "3D Pie.lvclass"=w283) -> (w287:T4)
          }
          frame "USER_RENDER_WINDOW" {
            n81 = Unbundle By Name(w324) -> ("Control Ref Queue"=w323:T5)
            n82 = call <vilib>:"Render Window Open.vi"("Control Ref Queue"=w323, "Object Cluster In"=w322) -> ("Object Cluster Out"=w321:T17)  [unwired: 3 in, 6 out]
          }
          frame "USER_EXPORT_IMAGE" {
            n83 = Unbundle By Name(w331) -> ("Control Ref Queue"=w330:T5)
            n84 = call <vilib>:"Image File Dialog.vi"("Control Ref Queue"=w330) -> ()  [unwired: 2 in, 9 out]
          }
          frame "USER_PRINT_IMAGE" {
            n85 = Unbundle By Name(w338) -> ("Control Ref Queue"=w341:T5)
            n86 = call <vilib>:"Image to Printer.vi"("Control Ref Queue"=w341) -> ()  [unwired: 1 in, 10 out]
          }
          frame "USER_PROJECTION_VISIBLE" {
            w355 = T18 1 items=["Attribute", "Show/Hide", "Cursor Move", "Zoom", "Mouse Drag", "XY Projection", "YZ Projection", "XZ Projection", "3D Projection", "Active Plot", "Scale"] ("Global String")
            n87 = Unbundle By Name(w359) -> ("3D Pie.lvclass"=w363:refnum<class "3D Pie.lvclass">, "Control Ref Queue"=w346:T5)
            n88 = call <vilib>:"Read Property.vi"("3D Plot.lvclass in"=w363) -> ("error out"=w348:errorcluster, "Property Cluster"=w361:T19, "3D Plot.lvclass out"=w362:refnum<class "3D Pie.lvclass">)  [unwired: 1 in, 7 out]
            n89 = Unbundle By Name(w361) -> ("Appearance Property.Visibility.Projection Palette"=w365:bool)
            n90 = Not(x=w365) -> (.not. x?=w352:bool)
            n91 = Bundle By Name(cluster=w361, "Appearance Property.Visibility.Projection Palette"=w352) -> (w360:T19)
            n92 = call <vilib>:"3DMathPlot Action String.vi"("Global String"=w355) -> ("String Out"=w354:string)  [unwired: 10 out]
            n93 = call <vilib>:"Write Property.vi"("error in (no error)"=w348, "Property Cluster"=w360, "3D Plot.lvclass in"=w362) -> ("error out"=w351:errorcluster, "3D Plot.lvclass out"=w350:refnum<class "3D Pie.lvclass">)  [unwired: 7 out]
            n94 = Bundle By Name(cluster=w367, "State Changed?"=TRUE ("Data Changed?"), "Action Name"=w354) -> (w366:T3)
            n95 = call <vilib>:"Update Palette with Legend.vi"("Control Ref Queue"=w346, "error in (no error)"=w351, "3D Plot.lvclass"=w350) -> ("Ignore the size change?"=w347:bool, "3D Plot.lvclass out"=w349:refnum<class "3D Pie.lvclass">)  [unwired: 7 out]
            n96 = Bundle By Name(cluster=w359, "3D Pie.lvclass"=w349) -> (w358:T4)
          }
          frame "USER_COLOR_RAMP_VISIBLE" {
            w377 = T18 1 items=["Attribute", "Show/Hide", "Cursor Move", "Zoom", "Mouse Drag", "XY Projection", "YZ Projection", "XZ Projection", "3D Projection", "Active Plot", "Scale"] ("Global String")
            n97 = Unbundle By Name(w385) -> ("3D Pie.lvclass"=w389:refnum<class "3D Pie.lvclass">, "Control Ref Queue"=w369:T5)
            n98 = call <vilib>:"Read Property.vi"("3D Plot.lvclass in"=w389) -> ("error out"=w371:errorcluster, "Property Cluster"=w388:T19, "3D Plot.lvclass out"=w375:refnum<class "3D Pie.lvclass">)  [unwired: 1 in, 7 out]
            n99 = Unbundle By Name(w388) -> ("Appearance Property.Visibility.Color Ramp Palette"=w390:bool)
            n100 = Not(x=w390) -> (.not. x?=w378:bool)
            n101 = Bundle By Name(cluster=w388, "Appearance Property.Visibility.Color Ramp Palette"=w378) -> (w387:T19)
            n102 = call <vilib>:"3DMathPlot Action String.vi"("Global String"=w377) -> ("String Out"=w386:string)  [unwired: 10 out]
            n103 = call <vilib>:"Write Property.vi"("error in (no error)"=w371, "Property Cluster"=w387, "3D Plot.lvclass in"=w375) -> ("error out"=w374:errorcluster, "3D Plot.lvclass out"=w373:refnum<class "3D Pie.lvclass">)  [unwired: 7 out]
            n104 = Bundle By Name(cluster=w380, "State Changed?"=TRUE ("Data Changed?"), "Action Name"=w386) -> (w379:T3)
            n105 = call <vilib>:"Update Palette with Legend.vi"("Control Ref Queue"=w369, "error in (no error)"=w374, "3D Plot.lvclass"=w373) -> ("Ignore the size change?"=w370:bool, "3D Plot.lvclass out"=w372:refnum<class "3D Pie.lvclass">)  [unwired: 7 out]
            n106 = Bundle By Name(cluster=w385, "3D Pie.lvclass"=w372) -> (w384:T4)
          }
        }
      }
      event "3D Picture Control": Mouse Down {
        n107 = event-data() -> ("PlatMods.Shift"=w412:bool, "Button"=w393:u16, "PlatMods.Ctrl"=w394:bool)  [unwired: 1 out]
        n108 = call <vilib>:"Check Right Click.vi"("Ctrl"=w394, "Button"=w393) -> ("Right Click?"=w392:bool)  [unwired: 9 out]
        n109 = case shown="False" w392 {
          tunnel: w412 -> [_ w445]
          tunnel: w411 -> [w424 w442]
          tunnel: w407 -> [_ w444]
          tunnel: [w424 w425] -> w402
          tunnel: [w423 w440] -> w399
          tunnel: w408 -> [w423 w439]
          tunnel: w406 -> [w422 w438]
          tunnel: [w422 w437] -> w398
          tunnel: w405 -> [w421 w435]
          tunnel: [w421 w435] -> w397
          tunnel: [w420 w436] -> w395
          tunnel: w403 -> [w420 w434]
          tunnel: [w419 w433] -> w396
          tunnel: w404 -> [w419 w432]
          tunnel: w410 -> [w417 w429]
          tunnel: w409 -> [w418 w428]
          tunnel: [w418 w427] -> w400
          tunnel: [w417 w426] -> w401
          frame True {
          }
          frame False {
            n110 = Unbundle By Name(w444) -> ("3D Pie.lvclass"=w443:refnum<class "3D Pie.lvclass">, "Control Ref Queue"=w431:T5)
            n111 = call <vilib>:"Read Property.vi"("3D Plot.lvclass in"=w443) -> ("Property Cluster"=w441:T19, "3D Plot.lvclass out"=w430:refnum<class "3D Pie.lvclass">)  [unwired: 1 in, 8 out]
            n112 = case shown="False" w435 {
              selector: w435 -> [_ w481]
              tunnel: w445 -> [w455 _]
              tunnel: w441 -> [w458 w484]
              tunnel: w442 -> [w463 w477]
              tunnel: [w455 w482] -> w440
              tunnel: w439 -> [_ w482]
              tunnel: w438 -> [w457 _]
              tunnel: [w457 w481] -> w437
              tunnel: [w456 w483] -> w436
              tunnel: w434 -> [w456 _]
              tunnel: [w454 w480] -> w433
              tunnel: w432 -> [_ w480]
              tunnel: w431 -> [w452 _]
              tunnel: w430 -> [w451 _]
              tunnel: w429 -> [w450 w478]
              tunnel: w428 -> [w449 w479]
              tunnel: [w448 w479] -> w427
              tunnel: [w447 w478] -> w426
              tunnel: [w446 w477] -> w425
              frame False {
                n113 = Unbundle By Name(w458) -> ("Graph Property.General Property.Fast Draw?"=w461:bool, "Graph Property.View Property.View Direction"=w462:T13, "Graph Property.View Property.User Defined View Direction.View Distance"=w454:sgl)
                n114 = Equal?(x=w462, y=T13."User Defined") -> (x = y?=w460:bool)
                n115 = And(x=w461, y=w460) -> (x .and. y?=w459:bool)
                n116 = case shown="True" w459 {
                  tunnel: w463 -> [w464 w475]
                  tunnel: w452 -> [_ w474]
                  tunnel: w451 -> [_ w473]
                  tunnel: w450 -> [w465 w472]
                  tunnel: w449 -> [w466 w471]
                  tunnel: [w466 w469] -> w448
                  tunnel: [w465 w468] -> w447
                  tunnel: [w464 w467] -> w446
                  frame False {
                  }
                  frame True {
                    # "Update the Fast Draw and display it."
                    n117 = call <vilib>:"Update Scene Object.vi"("Action"=T12 {"Light Action"=enum."Nothing", "Axis Action"=enum."Nothing", "Plot Action"=enum."Nothing", "Cursor Action"=enum."Nothing", "Fast Draw Action"=enum."Update"}, "Control Ref Queue"=w474, "Multiplot Representation In"=w471, "Object Cluster In"=w475, "Actual Transform In"=w472, "3D Plot.lvclass in"=w473) -> ("Object Cluster Out"=w467:T17, "Actual Transform Out"=w468:T10, "Multiplot Representation Out"=w469:T14)  [unwired: 1 in, 2 out]
                    n118 = Unbundle By Name(w467) -> ("Fast Root Scene Object"=w476:refnum<vi>)
                    n119 = local write "3D Picture Control"(w476) -> ()
                  }
                }
              }
              frame True {
                n120 = Unbundle By Name(w484) -> ("Cursor Property Array"=w483:T35)
              }
            }
          }
        }
      }
      event "3D Picture Control": Mouse Up {
        w491 = FALSE
        n121 = event-data() -> ("Button"=w496:u16)  [unwired: 1 out]
        n122 = case shown="1" w496 {
          tunnel: w499 -> [w507 w542]
          tunnel: w502 -> [w508 w524]
          tunnel: [w506 w532] -> w497
          tunnel: [w508 w529] -> w501
          tunnel: [w507 w541] -> w498
          tunnel: w495 -> [_ w539]
          tunnel: w494 -> [_ w538]
          tunnel: w493 -> [_ w534]
          tunnel: w500 -> [w506 w533]
          tunnel: w490 -> [w505 w518]
          tunnel: [w505 w519] -> w489
          tunnel: w488 -> [w504 w522]
          tunnel: [w504 w520] -> w487
          tunnel: w485 -> [_ w527]
          frame 0, Default {
          }
          frame 1 {
            n123 = Build Array(w539, w538) -> (w537:bool[])
            n124 = Unbundle By Name(w533) -> ("3D Pie.lvclass"=w516:refnum<class "3D Pie.lvclass">, "Control Ref Queue"=w523:T5)
            n125 = Boolean Array To Number(Boolean array=w537) -> (number=w536:u32)
            n126 = call <vilib>:"Read Property.vi"("3D Plot.lvclass in"=w516) -> ("error out"=w510:errorcluster, "Property Cluster"=w513:T19, "3D Plot.lvclass out"=w517:refnum<class "3D Pie.lvclass">)  [unwired: 1 in, 7 out]
            n127 = case shown="0, Default" w536 {
              tunnel: [w550 w556 w561] -> w540
              tunnel: [w545 TRUE ("State Changed?") TRUE ("State Changed?")] -> w535
              tunnel: w534 -> [_ _ w563]
              tunnel: w523 -> [w548 _ _]
              tunnel: w527 -> [_ w554 _]
              tunnel: w513 -> [w546 w553 w560]
              tunnel: [w547 w552 w559] -> w512
              tunnel: w510 -> [w544 w551 w558]
              tunnel: [w543 w551 w558] -> w509
              frame 0, Default {
                w549 = T18 4 items=["Attribute", "Show/Hide", "Cursor Move", "Zoom", "Mouse Drag", "XY Projection", "YZ Projection", "XZ Projection", "3D Projection", "Active Plot", "Scale"] ("Global String")
                n128 = call <vilib>:"Get Latitude & Longitude.vi"("Control Ref Queue"=w548, "error in (no error)"=w544, "Property Cluster in"=w546) -> ("error out"=w543:errorcluster, "State Changed?"=w545:bool, "Property Cluster out"=w547:T19)  [unwired: 6 out]
                n129 = call <vilib>:"3DMathPlot Action String.vi"("Global String"=w549) -> ("String Out"=w550:string)  [unwired: 10 out]
              }
              frame 1 {
                w555 = T18 3 items=["Attribute", "Show/Hide", "Cursor Move", "Zoom", "Mouse Drag", "XY Projection", "YZ Projection", "XZ Projection", "3D Projection", "Active Plot", "Scale"] ("Global String")
                n130 = Bundle By Name(cluster=w553, "Graph Property.View Property.User Defined View Direction.View Distance"=w554) -> (w552:T19)
                n131 = call <vilib>:"3DMathPlot Action String.vi"("Global String"=w555) -> ("String Out"=w556:string)  [unwired: 10 out]
              }
              frame 2 {
                w562 = T18 2 items=["Attribute", "Show/Hide", "Cursor Move", "Zoom", "Mouse Drag", "XY Projection", "YZ Projection", "XZ Projection", "3D Projection", "Active Plot", "Scale"] ("Global String")
                n132 = Bundle By Name(cluster=w560, "Cursor Property Array"=w563) -> (w559:T19)
                n133 = call <vilib>:"3DMathPlot Action String.vi"("Global String"=w562) -> ("String Out"=w561:string)  [unwired: 10 out]
              }
            }
            n134 = call <vilib>:"Write Property.vi"("error in (no error)"=w509, "Property Cluster"=w512, "3D Plot.lvclass in"=w517) -> ("error out"=w514:errorcluster, "3D Plot.lvclass out"=w515:refnum<class "3D Pie.lvclass">)  [unwired: 7 out]
            n135 = call <vilib>:"Scene Settings.vi"("Control Ref Queue"=w523, "error in (no error)"=w514, "Actual Transform In"=w522, "3D Plot.lvclass in"=w515) -> ("error out"=w526:errorcluster, "Actual Transform Out"=w521:T10, "3D Plot.lvclass out"=w525:refnum<class "3D Pie.lvclass">)  [unwired: 3 in, 2 out]
            n136 = call <vilib>:"Update Scene Object.vi"("Action"=T12 {"Light Action"=enum."Nothing", "Axis Action"=enum."Nothing", "Plot Action"=enum."Nothing", "Cursor Action"=enum."Update", "Fast Draw Action"=enum."Nothing"}, "Control Ref Queue"=w523, "Multiplot Representation In"=w518, "error in (no error)"=w526, "Object Cluster In"=w524, "Actual Transform In"=w521, "3D Plot.lvclass in"=w525) -> ("error out"=w528:errorcluster, "Object Cluster Out"=w529:T17, "Actual Transform Out"=w520:T10, "3D Plot.lvclass out"=w511:refnum<class "3D Pie.lvclass">, "Multiplot Representation Out"=w519:T14)
            n137 = Unbundle By Name(w529) -> ("Root Scene Object"=w530:refnum<vi>)
            n138 = call <vilib>:"Render Window Redraw.vi"("Control Ref Queue"=w523, "error in (no error)"=w528) -> ()  [unwired: 1 in, 9 out]
            n139 = Bundle By Name(cluster=w542, "State Changed?"=w535, "Action Name"=w540) -> (w541:T3)
            n140 = local write "3D Picture Control"(w530) -> ()
            n141 = Bundle By Name(cluster=w533, "3D Pie.lvclass"=w511) -> (w532:T4)
          }
        }
      }
      event "3D Picture Control": Mouse Move {
        n142 = event-data() -> ("Coords"=w568:T46)  [unwired: 1 out]
        n143 = Unbundle By Name(w583) -> ("3D Pie.lvclass"=w567:refnum<class "3D Pie.lvclass">, "Control Ref Queue"=w570:T5)
        n144 = call <vilib>:"Plot Zoom.vi"("Control Ref Queue"=w570, "Zoom Mode"=w585, "3D Plot.lvclass in"=w567) -> ("error out"=w582:errorcluster, "Dup Ortho Zoom Mode"=w584:bool, "3D Plot.lvclass out"=w566:refnum<class "3D Pie.lvclass">, "View Distance Out"=w565:sgl)  [unwired: 2 in, 3 out]
        n145 = call <vilib>:"Cursor Move.vi"("3D Plot.lvclass in"=w566, "Coords"=w568, "Control Ref Queue"=w570, "Actual Transform In"=w572, "Object Cluster In"=w581, "Cursor ID In"=w579, "Tracking Cursor?"=w575, "error in (no error)"=w582, "Multiplot Represention"=w573) -> ("Object Cluster Out"=w580:T17, "Cursor ID"=w578:i32, "Drag Cursor?"=w574:bool, "Update Plot?"=w576:bool, "Cursor Property Array"=w577:T35, "error out"=w569:errorcluster)  [unwired: 1 out]
        n146 = case shown="True" w576 {
          tunnel: w569 -> [_ w588]
          frame False {
          }
          frame True {
            n147 = invoke on="3D Picture Control" class="SceneGraphDisp (strict)" method="Redraw"(error in=w588) -> ()  [unwired: 2 in, 3 out]
          }
        }
      }
      event "Projection Palette.XY Projection": Value Change {
        w604 = T18 5 items=["Attribute", "Show/Hide", "Cursor Move", "Zoom", "Mouse Drag", "XY Projection", "YZ Projection", "XZ Projection", "3D Projection", "Active Plot", "Scale"] ("Global String")
        n148 = event-data() -> ("NewVal"=w590:bool)  [unwired: 1 out]
        n149 = Unbundle By Name(w609) -> ("3D Pie.lvclass"=w596:refnum<class "3D Pie.lvclass">, "Control Ref Queue"=w589:T5)
        n150 = call <vilib>:"View Direction Write.vi"("Control Ref Queue"=w589, "View Direction"=T13."Towards X-Y Plane", "3D Plot.lvclass in"=w596) -> ("error out"=w594:errorcluster, "3D Plot.lvclass out"=w595:refnum<class "3D Pie.lvclass">)  [unwired: 1 in, 6 out]
        n151 = call <vilib>:"Scene Settings.vi"("Control Ref Queue"=w589, "error in (no error)"=w594, "Actual Transform In"=w593, "3D Plot.lvclass in"=w595) -> ("error out"=w598:errorcluster, "Actual Transform Out"=w592:T10, "3D Plot.lvclass out"=w600:refnum<class "3D Pie.lvclass">)  [unwired: 3 in, 2 out]
        n152 = call <vilib>:"3DMathPlot Action String.vi"("Global String"=w604) -> ("String Out"=w605:string)  [unwired: 10 out]
        n153 = invoke on="3D Picture Control" class="SceneGraphDisp (strict)" method="Redraw"(error in=w598) -> (error out=w602:errorcluster)  [unwired: 2 in, 2 out]
        n154 = Bundle By Name(cluster=w608, "State Changed?"=w590, "Action Name"=w605) -> (w607:T3)
        n155 = call <vilib>:"Render Window Redraw.vi"("Control Ref Queue"=w589, "error in (no error)"=w602) -> ()  [unwired: 1 in, 9 out]
        n156 = Bundle By Name(cluster=w609, "3D Pie.lvclass"=w600) -> (w606:T4)
      }
      event "Projection Palette.XZ Projection": Value Change {
        w631 = T18 7 items=["Attribute", "Show/Hide", "Cursor Move", "Zoom", "Mouse Drag", "XY Projection", "YZ Projection", "XZ Projection", "3D Projection", "Active Plot", "Scale"] ("Global String")
        n157 = event-data() -> ("NewVal"=w617:bool)  [unwired: 1 out]
        n158 = Unbundle By Name(w636) -> ("3D Pie.lvclass"=w621:refnum<class "3D Pie.lvclass">, "Control Ref Queue"=w616:T5)
        n159 = call <vilib>:"View Direction Write.vi"("Control Ref Queue"=w616, "View Direction"=T13."Towards X-Z Plane", "3D Plot.lvclass in"=w621) -> ("error out"=w619:errorcluster, "3D Plot.lvclass out"=w620:refnum<class "3D Pie.lvclass">)  [unwired: 1 in, 6 out]
        n160 = call <vilib>:"Scene Settings.vi"("Control Ref Queue"=w616, "error in (no error)"=w619, "Actual Transform In"=w623, "3D Plot.lvclass in"=w620) -> ("error out"=w625:errorcluster, "Actual Transform Out"=w622:T10, "3D Plot.lvclass out"=w626:refnum<class "3D Pie.lvclass">)  [unwired: 4 in, 1 out]
        n161 = call <vilib>:"3DMathPlot Action String.vi"("Global String"=w631) -> ("String Out"=w632:string)  [unwired: 10 out]
        n162 = invoke on="3D Picture Control" class="SceneGraphDisp (strict)" method="Redraw"(error in=w625) -> (error out=w629:errorcluster)  [unwired: 2 in, 2 out]
        n163 = Bundle By Name(cluster=w634, "State Changed?"=w617, "Action Name"=w632) -> (w633:T3)
        n164 = call <vilib>:"Render Window Redraw.vi"("Control Ref Queue"=w616, "error in (no error)"=w629) -> ()  [unwired: 1 in, 9 out]
        n165 = Bundle By Name(cluster=w636, "3D Pie.lvclass"=w626) -> (w635:T4)
      }
      event "Projection Palette.YZ Projection": Value Change {
        w658 = T18 6 items=["Attribute", "Show/Hide", "Cursor Move", "Zoom", "Mouse Drag", "XY Projection", "YZ Projection", "XZ Projection", "3D Projection", "Active Plot", "Scale"] ("Global String")
        n166 = event-data() -> ("NewVal"=w644:bool)  [unwired: 1 out]
        n167 = Unbundle By Name(w663) -> ("3D Pie.lvclass"=w648:refnum<class "3D Pie.lvclass">, "Control Ref Queue"=w643:T5)
        n168 = call <vilib>:"View Direction Write.vi"("Control Ref Queue"=w643, "View Direction"=T13."Towards Y-Z Plane", "3D Plot.lvclass in"=w648) -> ("error out"=w646:errorcluster, "3D Plot.lvclass out"=w647:refnum<class "3D Pie.lvclass">)  [unwired: 1 in, 6 out]
        n169 = call <vilib>:"Scene Settings.vi"("Control Ref Queue"=w643, "error in (no error)"=w646, "Actual Transform In"=w650, "3D Plot.lvclass in"=w647) -> ("error out"=w652:errorcluster, "Actual Transform Out"=w649:T10, "3D Plot.lvclass out"=w654:refnum<class "3D Pie.lvclass">)  [unwired: 3 in, 2 out]
        n170 = call <vilib>:"3DMathPlot Action String.vi"("Global String"=w658) -> ("String Out"=w659:string)  [unwired: 10 out]
        n171 = invoke on="3D Picture Control" class="SceneGraphDisp (strict)" method="Redraw"(error in=w652) -> (error out=w656:errorcluster)  [unwired: 2 in, 2 out]
        n172 = Bundle By Name(cluster=w661, "State Changed?"=w644, "Action Name"=w659) -> (w660:T3)
        n173 = call <vilib>:"Render Window Redraw.vi"("Control Ref Queue"=w643, "error in (no error)"=w656) -> ()  [unwired: 1 in, 9 out]
        n174 = Bundle By Name(cluster=w663, "3D Pie.lvclass"=w654) -> (w662:T4)
      }
      event "Projection Palette.3D Projection": Value Change {
        w685 = T18 8 items=["Attribute", "Show/Hide", "Cursor Move", "Zoom", "Mouse Drag", "XY Projection", "YZ Projection", "XZ Projection", "3D Projection", "Active Plot", "Scale"] ("Global String")
        n175 = event-data() -> ("NewVal"=w671:bool)  [unwired: 1 out]
        n176 = Unbundle By Name(w690) -> ("3D Pie.lvclass"=w675:refnum<class "3D Pie.lvclass">, "Control Ref Queue"=w670:T5)
        n177 = call <vilib>:"View Direction Write.vi"("Control Ref Queue"=w670, "View Direction"=T13."User Defined", "3D Plot.lvclass in"=w675) -> ("error out"=w673:errorcluster, "3D Plot.lvclass out"=w674:refnum<class "3D Pie.lvclass">)  [unwired: 1 in, 6 out]
        n178 = call <vilib>:"Scene Settings.vi"("Control Ref Queue"=w670, "error in (no error)"=w673, "Actual Transform In"=w677, "3D Plot.lvclass in"=w674) -> ("error out"=w680:errorcluster, "Actual Transform Out"=w676:T10, "3D Plot.lvclass out"=w679:refnum<class "3D Pie.lvclass">)  [unwired: 3 in, 2 out]
        n179 = call <vilib>:"3DMathPlot Action String.vi"("Global String"=w685) -> ("String Out"=w686:string)  [unwired: 10 out]
        n180 = invoke on="3D Picture Control" class="SceneGraphDisp (strict)" method="Redraw"(error in=w680) -> (error out=w683:errorcluster)  [unwired: 2 in, 2 out]
        n181 = Bundle By Name(cluster=w688, "State Changed?"=w671, "Action Name"=w686) -> (w687:T3)
        n182 = call <vilib>:"Render Window Redraw.vi"("Control Ref Queue"=w670, "error in (no error)"=w683) -> ()  [unwired: 1 in, 9 out]
        n183 = Bundle By Name(cluster=w690, "3D Pie.lvclass"=w679) -> (w689:T4)
      }
      event "Color Ramp Palette.Active Plot": Value Change {
        w709 = T18 9 items=["Attribute", "Show/Hide", "Cursor Move", "Zoom", "Mouse Drag", "XY Projection", "YZ Projection", "XZ Projection", "3D Projection", "Active Plot", "Scale"] ("Global String")
        n184 = event-data() -> ("NewVal"=w712:i32)  [unwired: 1 out]
        n185 = Unbundle By Name(w714) -> ("3D Pie.lvclass"=w715:refnum<class "3D Pie.lvclass">, "Control Ref Queue"=w704:T5)
        n186 = call-dynamic "Write Active Plot.vi"("Active Plot"=w712, "3D Plot.lvclass in"=w715) -> ("error out"=w699:errorcluster, "3D Plot.lvclass out"=w700:refnum<class "3D Pie.lvclass">)  [unwired: 8 in]
        n187 = call <vilib>:"3DMathPlot Action String.vi"("Global String"=w709) -> ("String Out"=w710:string)  [unwired: 10 out]
        n188 = Bundle By Name(cluster=w708, "State Changed?"=TRUE ("Data Changed?"), "Action Name"=w710) -> (w707:T3)
        n189 = call-dynamic "Graph Color Legend.vi"("Control Ref Queue"=w704, "Multiplot Representation In"=w698, "error in (no error)"=w699, "3D Pie.lvclass in"=w700) -> ("3D Pie.lvclass out"=w706:refnum<class "3D Pie.lvclass">, "Multiplot Representation Out"=w697:T14)  [unwired: 2 in, 4 out]
        n190 = Bundle By Name(cluster=w714, "3D Pie.lvclass"=w706) -> (w713:T4)
      }
      event "Color Ramp Palette.Color Pair Array": Value Change {
        n191 = event-data() -> ("OldVal"=w742:cluster{"Color Box":u32, "String":string}[], "NewVal"=w739:cluster{"Color Box":u32, "String":string}[])  [unwired: 1 out]
        n192 = Equal?(x=w742, y=w739) -> (x = y?=w741:bool)
        n193 = case shown="False" w741 {
          tunnel: w737 -> [w769 w775]
          tunnel: [w767 w775] -> w732
          tunnel: w736 -> [w765 w773]
          tunnel: [w747 w773] -> w731
          tunnel: w740 -> [w764 w774]
          tunnel: w738 -> [w763 w772]
          tunnel: [w762 w772] -> w733
          tunnel: [w761 w776] -> w724
          tunnel: w734 -> [w760 w771]
          tunnel: [w759 w771] -> w735
          tunnel: w726 -> [w746 w776]
          tunnel: [w749 w774] -> w730
          tunnel: w739 -> [w754 _]
          frame False {
            w745 = T18 0 items=["Attribute", "Show/Hide", "Cursor Move", "Zoom", "Mouse Drag", "XY Projection", "YZ Projection", "XZ Projection", "3D Projection", "Active Plot", "Scale"] ("Global String")
            n194 = Unbundle By Name(w769) -> ("3D Pie.lvclass"=w757:refnum<class "3D Pie.lvclass">, "Control Ref Queue"=w750:T5)
            n195 = call-dynamic "Update Color Pair Array.vi"("Color Pair Array"=w754, "3D Pie.lvclass in"=w757) -> ("error out"=w755:errorcluster, "3D Pie.lvclass out"=w756:refnum<class "3D Pie.lvclass">)  [unwired: 1 in, 7 out]
            n196 = call <vilib>:"Update Scene Object.vi"("Action"=T12 {"Light Action"=enum."Nothing", "Axis Action"=enum."Nothing", "Plot Action"=enum."Update", "Cursor Action"=enum."Nothing", "Fast Draw Action"=enum."Nothing"}, "Control Ref Queue"=w750, "Multiplot Representation In"=w765, "error in (no error)"=w755, "Object Cluster In"=w763, "Actual Transform In"=w764, "3D Plot.lvclass in"=w756) -> ("error out"=w766:errorcluster, "Object Cluster Out"=w762:T17, "Actual Transform Out"=w749:T10, "3D Plot.lvclass out"=w770:refnum<class "3D Pie.lvclass">, "Multiplot Representation Out"=w748:T14)
            n197 = call <vilib>:"3DMathPlot Action String.vi"("Global String"=w745) -> ("String Out"=w744:string)  [unwired: 10 out]
            n198 = Bundle By Name(cluster=w760, "State Changed?"=TRUE, "Action Name"=w744) -> (w759:T3)
            n199 = call-dynamic "Graph Color Legend.vi"("Control Ref Queue"=w750, "Multiplot Representation In"=w748, "error in (no error)"=w766, "Former Ignore States"=w746, "3D Pie.lvclass in"=w770) -> ("error out"=w752:errorcluster, "Ignore the size change?"=w761:bool, "3D Pie.lvclass out"=w768:refnum<class "3D Pie.lvclass">, "Multiplot Representation Out"=w747:T14)  [unwired: 1 in, 2 out]
            n200 = call <vilib>:"Render Window Redraw.vi"("Control Ref Queue"=w750, "error in (no error)"=w752) -> ("error out"=w751:errorcluster)  [unwired: 1 in, 8 out]
            n201 = invoke on="3D Picture Control" class="SceneGraphDisp (strict)" method="Redraw"(error in=w751) -> ()  [unwired: 2 in, 3 out]
            n202 = Bundle By Name(cluster=w769, "3D Pie.lvclass"=w768) -> (w767:T4)
          }
          frame True {
          }
        }
      }
      event "XY Graph": Scale Range Change {
        w792 = T18 10 items=["Attribute", "Show/Hide", "Cursor Move", "Zoom", "Mouse Drag", "XY Projection", "YZ Projection", "XZ Projection", "3D Projection", "Active Plot", "Scale"] ("Global String")
        n203 = event-data() -> ("NewRange"=w803:T47, "Kind"=w802:enum16{"X-Scale", "Y-Scale", "Z-Scale"})  [unwired: 1 out]
        n204 = Unbundle By Name(w800) -> ("3D Pie.lvclass"=w801:refnum<class "3D Pie.lvclass">, "Control Ref Queue"=w785:T5)
        n205 = call <vilib>:"Transform Cluster Update.vi"("Axis"=w802, "NewRange"=w803, "Multiplot Representation In"=w778, "Actual Transform In"=w781, "3D Plot in"=w801) -> ("error out"=w787:errorcluster, "Actual Transform Out"=w780:T10, "3D Plot out"=w788:refnum<class "3D Pie.lvclass">, "Multiplot Representation Out"=w779:T14)  [unwired: 1 in, 2 out]
        n206 = call <vilib>:"Update Scene Object.vi"("Action"=T12 {"Light Action"=enum."Nothing", "Axis Action"=enum."Update", "Plot Action"=enum."Update", "Cursor Action"=enum."Update", "Fast Draw Action"=enum."Nothing"}, "Control Ref Queue"=w785, "Multiplot Representation In"=w779, "error in (no error)"=w787, "Object Cluster In"=w794, "Actual Transform In"=w780, "3D Plot.lvclass in"=w788) -> ("error out"=w789:errorcluster, "Object Cluster Out"=w795:T17, "Actual Transform Out"=w783:T10, "3D Plot.lvclass out"=w777:refnum<class "3D Pie.lvclass">, "Multiplot Representation Out"=w782:T14)
        n207 = invoke on="3D Picture Control" class="SceneGraphDisp (strict)" method="Redraw"(error in=w789) -> (error out=w786:errorcluster)  [unwired: 2 in, 2 out]
        n208 = call <vilib>:"3DMathPlot Action String.vi"("Global String"=w792) -> ("String Out"=w793:string)  [unwired: 10 out]
        n209 = call <vilib>:"Render Window Redraw.vi"("Control Ref Queue"=w785, "error in (no error)"=w786) -> ()  [unwired: 1 in, 9 out]
        n210 = Bundle By Name(cluster=w797, "State Changed?"=TRUE ("Data Changed?"), "Action Name"=w793) -> (w796:T3)
        n211 = Bundle By Name(cluster=w800, "3D Pie.lvclass"=w777) -> (w799:T4)
      }
      event Panel Resize {
        n212 = event-data() -> ()  [unwired: 2 out]
        n213 = First Call?() -> (First Call?: T/F=w812:bool)
        n214 = Or(x=w812, y=w811) -> (x .or. y?=w810:bool)
        n215 = case shown="False" w810 {
          tunnel: w818 -> [w831 w833]
          tunnel: [w830 w833] -> w817
          frame False {
            n216 = Unbundle By Name(w831) -> ("3D Pie.lvclass"=w832:refnum<class "3D Pie.lvclass">, "Control Ref Queue"=w829:T5)
            n217 = call <vilib>:"Panel Resize.vi"("Control Ref Queue"=w829, "3D Plot.lvclass"=w832) -> ("error out"=w827:errorcluster, "3D Plot.lvclass out"=w828:refnum<class "3D Pie.lvclass">)  [unwired: 3 in, 5 out]
            n218 = invoke on="3D Picture Control" class="SceneGraphDisp (strict)" method="Redraw"(error in=w827) -> ()  [unwired: 2 in, 3 out]
            n219 = Bundle By Name(cluster=w831, "3D Pie.lvclass"=w828) -> (w830:T4)
          }
          frame True {
          }
        }
      }
    }
  }
  "Display State Out" <- w4
  "Data Out" <- w5
  "Action" <- w3
